vi "Forebrain.vi"() -> ()   [LabVIEW 2012]
doc: "This VI contrains the Forebrain within the Olin Robot Architecture. It must be run first to load the appropriate mission definition files. It contains a finite state machine built around a tabbed Operator interface that will guide an operator through the startup, run shutdown mission sequence. After running it, run the Midbrain and Hindbrain VIS."
panel:
  out "current MDF":T1(array[cluster])=[{"Status"=enum."Current", "x"=516.0, "y"=516.0, "z"=0.0, "Vel"=3.0, "Dwell Time"=0.0, "BehCom"=enum."Manual Mode", "X1"=0.0, "Y1"=0.0, "X2"=0.0, "Y2"=0.0}, {"Status"=enum."Future", "x"=0.0, "y"=0.0, "z"=0.0, "Vel"=0.0, "Dwell Time"=0.0, "BehCom"=enum."Tug Off", "X1"=0.0, "Y1"=0.0, "X2"=0.0, "Y2"=0.0}, {"Status"=enum."Future", "x"=0.0, "y"=0.0, "z"=0.0, "Vel"=0.0, "Dwell Time"=0.0, "BehCom"=enum."Tug Off", "X1"=0.0, "Y1"=0.0, "X2"=0.0, "Y2"=0.0}, {"Status"=enum."Future", "x"=0.0, "y"=0.0, "z"=0.0, "Vel"=0.0, "Dwell Time"=0.0, "BehCom"=enum."Tug Off", "X1"=0.0, "Y1"=0.0, "X2"=0.0, "Y2"=0.0}, {"Status"=enum."Future", "x"=0.0, "y"=0.0, "z"=0.0, "Vel"=0.0, "Dwell Time"=0.0, "BehCom"=enum."Tug Off", "X1"=0.0, "Y1"=0.0, "X2"=0.0, "Y2"=0.0}, {"Status"=enum."Future", "x"=0.0, "y"=0.0, "z"=0.0, "Vel"=0.0, "Dwell Time"=0.0, "BehCom"=enum."Tug Off", "X1"=0.0, "Y1"=0.0, "X2"=0.0, "Y2"=0.0}, {"Status"=enum."Future", "x"=0.0, "y"=0.0, "z"=0.0, "Vel"=0.0, "Dwell Time"=0.0, "BehCom"=enum."Tug Off", "X1"=0.0, "Y1"=0.0, "X2"=0.0, "Y2"=0.0}, {"Status"=enum."Future", "x"=0.0, "y"=0.0, "z"=0.0, "Vel"=0.0, "Dwell Time"=0.0, "BehCom"=enum."Tug Off", "X1"=0.0, "Y1"=0.0, "X2"=0.0, "Y2"=0.0}, {"Status"=enum."Future", "x"=0.0, "y"=0.0, "z"=0.0, "Vel"=0.0, "Dwell Time"=0.0, "BehCom"=enum."Tug Off", "X1"=0.0, "Y1"=0.0, "X2"=0.0, "Y2"=0.0}, {"Status"=enum."Future", "x"=0.0, "y"=0.0, "z"=0.0, "Vel"=0.0, "Dwell Time"=0.0, "BehCom"=enum."Tug Off", "X1"=0.0, "Y1"=0.0, "X2"=0.0, "Y2"=0.0}, {"Status"=enum."Future", "x"=0.0, "y"=0.0, "z"=0.0, "Vel"=0.0, "Dwell Time"=0.0, "BehCom"=enum."Tug Off", "X1"=0.0, "Y1"=0.0, "X2"=0.0, "Y2"=0.0}, {"Status"=enum."Future", "x"=0.0, "y"=0.0, "z"=0.0, "Vel"=0.0, "Dwell Time"=0.0, "BehCom"=enum."Tug Off", "X1"=0.0, "Y1"=0.0, "X2"=0.0, "Y2"=0.0}, {"Status"=enum."Future", "x"=0.0, "y"=0.0, "z"=0.0, "Vel"=0.0, "Dwell Time"=0.0, "BehCom"=enum."Tug Off", "X1"=0.0, "Y1"=0.0, "X2"=0.0, "Y2"=0.0}, {"Status"=enum."Future", "x"=0.0, "y"=0.0, "z"=0.0, "Vel"=0.0, "Dwell Time"=0.0, "BehCom"=enum."Tug Off", "X1"=0.0, "Y1"=0.0, "X2"=0.0, "Y2"=0.0}, {"Status"=enum."Future", "x"=0.0, "y"=0.0, "z"=0.0, "Vel"=0.0, "Dwell Time"=0.0, "BehCom"=enum."Tug Off", "X1"=0.0, "Y1"=0.0, "X2"=0.0, "Y2"=0.0}, {"Status"=enum."Future", "x"=0.0, "y"=0.0, "z"=0.0, "Vel"=0.0, "Dwell Time"=0.0, "BehCom"=enum."Tug Off", "X1"=0.0, "Y1"=0.0, "X2"=0.0, "Y2"=0.0}, {"Status"=enum."Future", "x"=0.0, "y"=0.0, "z"=0.0, "Vel"=0.0, "Dwell Time"=0.0, "BehCom"=enum."Tug Off", "X1"=0.0, "Y1"=0.0, "X2"=0.0, "Y2"=0.0}, {"Status"=enum."Future", "x"=0.0, "y"=0.0, "z"=0.0, "Vel"=0.0, "Dwell Time"=0.0, "BehCom"=enum."Tug Off", "X1"=0.0, "Y1"=0.0, "X2"=0.0, "Y2"=0.0}, {"Status"=enum."Future", "x"=0.0, "y"=0.0, "z"=0.0, "Vel"=0.0, "Dwell Time"=0.0, "BehCom"=enum."Tug Off", "X1"=0.0, "Y1"=0.0, "X2"=0.0, "Y2"=0.0}, {"Status"=enum."Future", "x"=0.0, "y"=0.0, "z"=0.0, "Vel"=0.0, "Dwell Time"=0.0, "BehCom"=enum."Tug Off", "X1"=0.0, "Y1"=0.0, "X2"=0.0, "Y2"=0.0}, {"Status"=enum."Future", "x"=0.0, "y"=0.0, "z"=0.0, "Vel"=0.0, "Dwell Time"=0.0, "BehCom"=enum."Tug Off", "X1"=0.0, "Y1"=0.0, "X2"=0.0, "Y2"=0.0}, {"Status"=enum."Future", "x"=0.0, "y"=0.0, "z"=0.0, "Vel"=0.0, "Dwell Time"=0.0, "BehCom"=enum."Tug Off", "X1"=0.0, "Y1"=0.0, "X2"=0.0, "Y2"=0.0}, {"Status"=enum."Future", "x"=0.0, "y"=0.0, "z"=0.0, "Vel"=0.0, "Dwell Time"=0.0, "BehCom"=enum."Tug Off", "X1"=0.0, "Y1"=0.0, "X2"=0.0, "Y2"=0.0}, {"Status"=enum."Future", "x"=0.0, "y"=0.0, "z"=0.0, "Vel"=0.0, "Dwell Time"=0.0, "BehCom"=enum."Tug Off", "X1"=0.0, "Y1"=0.0, "X2"=0.0, "Y2"=0.0}, {"Status"=enum."Future", "x"=0.0, "y"=0.0, "z"=0.0, "Vel"=0.0, "Dwell Time"=0.0, "BehCom"=enum."Tug Off", "X1"=0.0, "Y1"=0.0, "X2"=0.0, "Y2"=0.0}, {"Status"=enum."Future", "x"=0.0, "y"=0.0, "z"=0.0, "Vel"=0.0, "Dwell Time"=0.0, "BehCom"=enum."Tug Off", "X1"=0.0, "Y1"=0.0, "X2"=0.0, "Y2"=0.0}, {"Status"=enum."Future", "x"=0.0, "y"=0.0, "z"=0.0, "Vel"=0.0, "Dwell Time"=0.0, "BehCom"=enum."Tug Off", "X1"=0.0, "Y1"=0.0, "X2"=0.0, "Y2"=0.0}, {"Status"=enum."Future", "x"=0.0, "y"=0.0, "z"=0.0, "Vel"=0.0, "Dwell Time"=0.0, "BehCom"=enum."Tug Off", "X1"=0.0, "Y1"=0.0, "X2"=0.0, "Y2"=0.0}, {"Status"=enum."Future", "x"=0.0, "y"=0.0, "z"=0.0, "Vel"=0.0, "Dwell Time"=0.0, "BehCom"=enum."Tug Off", "X1"=0.0, "Y1"=0.0, "X2"=0.0, "Y2"=0.0}, {"Status"=enum."Future", "x"=0.0, "y"=0.0, "z"=0.0, "Vel"=0.0, "Dwell Time"=0.0, "BehCom"=enum."Tug Off", "X1"=0.0, "Y1"=0.0, "X2"=0.0, "Y2"=0.0}]
  out "Original MDF":T1(array[cluster])=[{"Status"=enum."Current", "x"=516.0, "y"=516.0, "z"=0.0, "Vel"=3.0, "Dwell Time"=0.0, "BehCom"=enum."Manual Mode", "X1"=0.0, "Y1"=0.0, "X2"=0.0, "Y2"=0.0}, {"Status"=enum."Future", "x"=0.0, "y"=0.0, "z"=0.0, "Vel"=0.0, "Dwell Time"=0.0, "BehCom"=enum."Tug Off", "X1"=0.0, "Y1"=0.0, "X2"=0.0, "Y2"=0.0}, {"Status"=enum."Future", "x"=0.0, "y"=0.0, "z"=0.0, "Vel"=0.0, "Dwell Time"=0.0, "BehCom"=enum."Tug Off", "X1"=0.0, "Y1"=0.0, "X2"=0.0, "Y2"=0.0}, {"Status"=enum."Future", "x"=0.0, "y"=0.0, "z"=0.0, "Vel"=0.0, "Dwell Time"=0.0, "BehCom"=enum."Tug Off", "X1"=0.0, "Y1"=0.0, "X2"=0.0, "Y2"=0.0}, {"Status"=enum."Future", "x"=0.0, "y"=0.0, "z"=0.0, "Vel"=0.0, "Dwell Time"=0.0, "BehCom"=enum."Tug Off", "X1"=0.0, "Y1"=0.0, "X2"=0.0, "Y2"=0.0}, {"Status"=enum."Future", "x"=0.0, "y"=0.0, "z"=0.0, "Vel"=0.0, "Dwell Time"=0.0, "BehCom"=enum."Tug Off", "X1"=0.0, "Y1"=0.0, "X2"=0.0, "Y2"=0.0}, {"Status"=enum."Future", "x"=0.0, "y"=0.0, "z"=0.0, "Vel"=0.0, "Dwell Time"=0.0, "BehCom"=enum."Tug Off", "X1"=0.0, "Y1"=0.0, "X2"=0.0, "Y2"=0.0}, {"Status"=enum."Future", "x"=0.0, "y"=0.0, "z"=0.0, "Vel"=0.0, "Dwell Time"=0.0, "BehCom"=enum."Tug Off", "X1"=0.0, "Y1"=0.0, "X2"=0.0, "Y2"=0.0}, {"Status"=enum."Future", "x"=0.0, "y"=0.0, "z"=0.0, "Vel"=0.0, "Dwell Time"=0.0, "BehCom"=enum."Tug Off", "X1"=0.0, "Y1"=0.0, "X2"=0.0, "Y2"=0.0}, {"Status"=enum."Future", "x"=0.0, "y"=0.0, "z"=0.0, "Vel"=0.0, "Dwell Time"=0.0, "BehCom"=enum."Tug Off", "X1"=0.0, "Y1"=0.0, "X2"=0.0, "Y2"=0.0}, {"Status"=enum."Future", "x"=0.0, "y"=0.0, "z"=0.0, "Vel"=0.0, "Dwell Time"=0.0, "BehCom"=enum."Tug Off", "X1"=0.0, "Y1"=0.0, "X2"=0.0, "Y2"=0.0}, {"Status"=enum."Future", "x"=0.0, "y"=0.0, "z"=0.0, "Vel"=0.0, "Dwell Time"=0.0, "BehCom"=enum."Tug Off", "X1"=0.0, "Y1"=0.0, "X2"=0.0, "Y2"=0.0}, {"Status"=enum."Future", "x"=0.0, "y"=0.0, "z"=0.0, "Vel"=0.0, "Dwell Time"=0.0, "BehCom"=enum."Tug Off", "X1"=0.0, "Y1"=0.0, "X2"=0.0, "Y2"=0.0}, {"Status"=enum."Future", "x"=0.0, "y"=0.0, "z"=0.0, "Vel"=0.0, "Dwell Time"=0.0, "BehCom"=enum."Tug Off", "X1"=0.0, "Y1"=0.0, "X2"=0.0, "Y2"=0.0}, {"Status"=enum."Future", "x"=0.0, "y"=0.0, "z"=0.0, "Vel"=0.0, "Dwell Time"=0.0, "BehCom"=enum."Tug Off", "X1"=0.0, "Y1"=0.0, "X2"=0.0, "Y2"=0.0}, {"Status"=enum."Future", "x"=0.0, "y"=0.0, "z"=0.0, "Vel"=0.0, "Dwell Time"=0.0, "BehCom"=enum."Tug Off", "X1"=0.0, "Y1"=0.0, "X2"=0.0, "Y2"=0.0}, {"Status"=enum."Future", "x"=0.0, "y"=0.0, "z"=0.0, "Vel"=0.0, "Dwell Time"=0.0, "BehCom"=enum."Tug Off", "X1"=0.0, "Y1"=0.0, "X2"=0.0, "Y2"=0.0}, {"Status"=enum."Future", "x"=0.0, "y"=0.0, "z"=0.0, "Vel"=0.0, "Dwell Time"=0.0, "BehCom"=enum."Tug Off", "X1"=0.0, "Y1"=0.0, "X2"=0.0, "Y2"=0.0}, {"Status"=enum."Future", "x"=0.0, "y"=0.0, "z"=0.0, "Vel"=0.0, "Dwell Time"=0.0, "BehCom"=enum."Tug Off", "X1"=0.0, "Y1"=0.0, "X2"=0.0, "Y2"=0.0}, {"Status"=enum."Future", "x"=0.0, "y"=0.0, "z"=0.0, "Vel"=0.0, "Dwell Time"=0.0, "BehCom"=enum."Tug Off", "X1"=0.0, "Y1"=0.0, "X2"=0.0, "Y2"=0.0}, {"Status"=enum."Future", "x"=0.0, "y"=0.0, "z"=0.0, "Vel"=0.0, "Dwell Time"=0.0, "BehCom"=enum."Tug Off", "X1"=0.0, "Y1"=0.0, "X2"=0.0, "Y2"=0.0}, {"Status"=enum."Future", "x"=0.0, "y"=0.0, "z"=0.0, "Vel"=0.0, "Dwell Time"=0.0, "BehCom"=enum."Tug Off", "X1"=0.0, "Y1"=0.0, "X2"=0.0, "Y2"=0.0}, {"Status"=enum."Future", "x"=0.0, "y"=0.0, "z"=0.0, "Vel"=0.0, "Dwell Time"=0.0, "BehCom"=enum."Tug Off", "X1"=0.0, "Y1"=0.0, "X2"=0.0, "Y2"=0.0}, {"Status"=enum."Future", "x"=0.0, "y"=0.0, "z"=0.0, "Vel"=0.0, "Dwell Time"=0.0, "BehCom"=enum."Tug Off", "X1"=0.0, "Y1"=0.0, "X2"=0.0, "Y2"=0.0}, {"Status"=enum."Future", "x"=0.0, "y"=0.0, "z"=0.0, "Vel"=0.0, "Dwell Time"=0.0, "BehCom"=enum."Tug Off", "X1"=0.0, "Y1"=0.0, "X2"=0.0, "Y2"=0.0}, {"Status"=enum."Future", "x"=0.0, "y"=0.0, "z"=0.0, "Vel"=0.0, "Dwell Time"=0.0, "BehCom"=enum."Tug Off", "X1"=0.0, "Y1"=0.0, "X2"=0.0, "Y2"=0.0}, {"Status"=enum."Future", "x"=0.0, "y"=0.0, "z"=0.0, "Vel"=0.0, "Dwell Time"=0.0, "BehCom"=enum."Tug Off", "X1"=0.0, "Y1"=0.0, "X2"=0.0, "Y2"=0.0}, {"Status"=enum."Future", "x"=0.0, "y"=0.0, "z"=0.0, "Vel"=0.0, "Dwell Time"=0.0, "BehCom"=enum."Tug Off", "X1"=0.0, "Y1"=0.0, "X2"=0.0, "Y2"=0.0}, {"Status"=enum."Future", "x"=0.0, "y"=0.0, "z"=0.0, "Vel"=0.0, "Dwell Time"=0.0, "BehCom"=enum."Tug Off", "X1"=0.0, "Y1"=0.0, "X2"=0.0, "Y2"=0.0}, {"Status"=enum."Future", "x"=0.0, "y"=0.0, "z"=0.0, "Vel"=0.0, "Dwell Time"=0.0, "BehCom"=enum."Tug Off", "X1"=0.0, "Y1"=0.0, "X2"=0.0, "Y2"=0.0}]
  out "No. of Waypoints":i32=30
  in  "A Midbrain?":bool
  in  "Manuel\nLocation":bool
  in  "Fake Heading":i32
  in  "Fake X":i32
  in  "Fake Y":i32
  out "return count":u32=11
  out "error out":errorcluster
  in  "error in 2":errorcluster
  out "Desired \nVelocity":i16
  out "Local\nHeading":i16
  out "Ycurrent":dbl=744.0 format="%#_3g"
  out "Xcurrent":dbl=683.0 format="%#_3g"
  out "Ystart":dbl=400.0
  out "Xstart":dbl=500.0
  in  "error in":errorcluster
  out "Robot Live":bool=TRUE
  in  "E-Stop":bool
  in  "Tab":T2(tab)=enum."PlanMission"
  out "MissionTime (Min)":dbl(knob)=1.6143843173980712 scale=0.0..10.0
  out "LidarDist":i16=800
  out "IR Index":i32
  out "BatteryLevel":dbl(slide)=7.0 scale=6.0..9.0
  out "String Received":string="{800,13,48520}<13,10,13>"
  out "Send String":string="[AGHBAAAAA]"
  in  "VISA resource name":refnum<visa-resource-name>="COM7"
  in  "Mode":i16=1 min=0 max=99 step=1
  in  "Desired Vel":i16(slide) scale=-9.0..9.0
  in  "Local Head":i16(slide) scale=-180.0..180.0
  out "StartMissionMap":picture
  out "MapDARCheck":picture
  in  "RunRobot":bool=TRUE
  in  "Tug letter":string="T"
  out "Tug X":i32=683
  out "Tug Y":i32=744
  out "Tug H":i32=220
  out "BS Time Out?":bool
  out "Buoy locations":cluster{"regular expression":string, i32, i32}[](array[cluster])=[{"regular expression"="A", 229, 772}, {"regular expression"="B", 828, 412}, {"regular expression"="C", 634, 873}, {"regular expression"="D", 229, 278}]
  out "Valid ?":bool
  out "Battery\nVolts":i16=7000
  out "Base Station data rec'd":string="$,G,-1,-1,-1,T,-1,-1,-1,P,-1,-1,-1,L,-1,-1,-1,A,229,772,B,828,412,C,634,873,D,229,278,S,23,43,27\r"
  out "udp rate":bool=TRUE
  out "CollisionWarning":bool
  out "DebugMapDAR":picture
  in  "MapDAR Control":T3={"NumberOfBeams"=180, "SensorRange"=500.0, "Noise (0.1 to 1)"=0.0} {"Noise (0.1 to 1)" min=0.0 max=1.0 step=0.1; "SensorRange" min=500.0 max=1500.0 step=100.0; "NumberOfBeams" min=36 max=360 step=2}
  out "MapDAR Data (r:pixel b:degrees)":cluster{"Range":dbl, "Bearing":dbl}[](array[cluster])
  in  "Stop DebugSENSE":bool
  out "MissionMap":picture
  out "Tug position":T4
  out "initialized MDF":T1(array[cluster])=[{"Status"=enum."Current", "x"=516.0, "y"=516.0, "z"=0.0, "Vel"=3.0, "Dwell Time"=0.0, "BehCom"=enum."Manual Mode", "X1"=0.0, "Y1"=0.0, "X2"=0.0, "Y2"=0.0}, {"Status"=enum."Future", "x"=0.0, "y"=0.0, "z"=0.0, "Vel"=0.0, "Dwell Time"=0.0, "BehCom"=enum."Tug Off", "X1"=0.0, "Y1"=0.0, "X2"=0.0, "Y2"=0.0}, {"Status"=enum."Future", "x"=0.0, "y"=0.0, "z"=0.0, "Vel"=0.0, "Dwell Time"=0.0, "BehCom"=enum."Tug Off", "X1"=0.0, "Y1"=0.0, "X2"=0.0, "Y2"=0.0}, {"Status"=enum."Future", "x"=0.0, "y"=0.0, "z"=0.0, "Vel"=0.0, "Dwell Time"=0.0, "BehCom"=enum."Tug Off", "X1"=0.0, "Y1"=0.0, "X2"=0.0, "Y2"=0.0}, {"Status"=enum."Future", "x"=0.0, "y"=0.0, "z"=0.0, "Vel"=0.0, "Dwell Time"=0.0, "BehCom"=enum."Tug Off", "X1"=0.0, "Y1"=0.0, "X2"=0.0, "Y2"=0.0}, {"Status"=enum."Future", "x"=0.0, "y"=0.0, "z"=0.0, "Vel"=0.0, "Dwell Time"=0.0, "BehCom"=enum."Tug Off", "X1"=0.0, "Y1"=0.0, "X2"=0.0, "Y2"=0.0}, {"Status"=enum."Future", "x"=0.0, "y"=0.0, "z"=0.0, "Vel"=0.0, "Dwell Time"=0.0, "BehCom"=enum."Tug Off", "X1"=0.0, "Y1"=0.0, "X2"=0.0, "Y2"=0.0}, {"Status"=enum."Future", "x"=0.0, "y"=0.0, "z"=0.0, "Vel"=0.0, "Dwell Time"=0.0, "BehCom"=enum."Tug Off", "X1"=0.0, "Y1"=0.0, "X2"=0.0, "Y2"=0.0}, {"Status"=enum."Future", "x"=0.0, "y"=0.0, "z"=0.0, "Vel"=0.0, "Dwell Time"=0.0, "BehCom"=enum."Tug Off", "X1"=0.0, "Y1"=0.0, "X2"=0.0, "Y2"=0.0}, {"Status"=enum."Future", "x"=0.0, "y"=0.0, "z"=0.0, "Vel"=0.0, "Dwell Time"=0.0, "BehCom"=enum."Tug Off", "X1"=0.0, "Y1"=0.0, "X2"=0.0, "Y2"=0.0}, {"Status"=enum."Future", "x"=0.0, "y"=0.0, "z"=0.0, "Vel"=0.0, "Dwell Time"=0.0, "BehCom"=enum."Tug Off", "X1"=0.0, "Y1"=0.0, "X2"=0.0, "Y2"=0.0}, {"Status"=enum."Future", "x"=0.0, "y"=0.0, "z"=0.0, "Vel"=0.0, "Dwell Time"=0.0, "BehCom"=enum."Tug Off", "X1"=0.0, "Y1"=0.0, "X2"=0.0, "Y2"=0.0}, {"Status"=enum."Future", "x"=0.0, "y"=0.0, "z"=0.0, "Vel"=0.0, "Dwell Time"=0.0, "BehCom"=enum."Tug Off", "X1"=0.0, "Y1"=0.0, "X2"=0.0, "Y2"=0.0}, {"Status"=enum."Future", "x"=0.0, "y"=0.0, "z"=0.0, "Vel"=0.0, "Dwell Time"=0.0, "BehCom"=enum."Tug Off", "X1"=0.0, "Y1"=0.0, "X2"=0.0, "Y2"=0.0}, {"Status"=enum."Future", "x"=0.0, "y"=0.0, "z"=0.0, "Vel"=0.0, "Dwell Time"=0.0, "BehCom"=enum."Tug Off", "X1"=0.0, "Y1"=0.0, "X2"=0.0, "Y2"=0.0}, {"Status"=enum."Future", "x"=0.0, "y"=0.0, "z"=0.0, "Vel"=0.0, "Dwell Time"=0.0, "BehCom"=enum."Tug Off", "X1"=0.0, "Y1"=0.0, "X2"=0.0, "Y2"=0.0}, {"Status"=enum."Future", "x"=0.0, "y"=0.0, "z"=0.0, "Vel"=0.0, "Dwell Time"=0.0, "BehCom"=enum."Tug Off", "X1"=0.0, "Y1"=0.0, "X2"=0.0, "Y2"=0.0}, {"Status"=enum."Future", "x"=0.0, "y"=0.0, "z"=0.0, "Vel"=0.0, "Dwell Time"=0.0, "BehCom"=enum."Tug Off", "X1"=0.0, "Y1"=0.0, "X2"=0.0, "Y2"=0.0}, {"Status"=enum."Future", "x"=0.0, "y"=0.0, "z"=0.0, "Vel"=0.0, "Dwell Time"=0.0, "BehCom"=enum."Tug Off", "X1"=0.0, "Y1"=0.0, "X2"=0.0, "Y2"=0.0}, {"Status"=enum."Future", "x"=0.0, "y"=0.0, "z"=0.0, "Vel"=0.0, "Dwell Time"=0.0, "BehCom"=enum."Tug Off", "X1"=0.0, "Y1"=0.0, "X2"=0.0, "Y2"=0.0}, {"Status"=enum."Future", "x"=0.0, "y"=0.0, "z"=0.0, "Vel"=0.0, "Dwell Time"=0.0, "BehCom"=enum."Tug Off", "X1"=0.0, "Y1"=0.0, "X2"=0.0, "Y2"=0.0}, {"Status"=enum."Future", "x"=0.0, "y"=0.0, "z"=0.0, "Vel"=0.0, "Dwell Time"=0.0, "BehCom"=enum."Tug Off", "X1"=0.0, "Y1"=0.0, "X2"=0.0, "Y2"=0.0}, {"Status"=enum."Future", "x"=0.0, "y"=0.0, "z"=0.0, "Vel"=0.0, "Dwell Time"=0.0, "BehCom"=enum."Tug Off", "X1"=0.0, "Y1"=0.0, "X2"=0.0, "Y2"=0.0}, {"Status"=enum."Future", "x"=0.0, "y"=0.0, "z"=0.0, "Vel"=0.0, "Dwell Time"=0.0, "BehCom"=enum."Tug Off", "X1"=0.0, "Y1"=0.0, "X2"=0.0, "Y2"=0.0}, {"Status"=enum."Future", "x"=0.0, "y"=0.0, "z"=0.0, "Vel"=0.0, "Dwell Time"=0.0, "BehCom"=enum."Tug Off", "X1"=0.0, "Y1"=0.0, "X2"=0.0, "Y2"=0.0}, {"Status"=enum."Future", "x"=0.0, "y"=0.0, "z"=0.0, "Vel"=0.0, "Dwell Time"=0.0, "BehCom"=enum."Tug Off", "X1"=0.0, "Y1"=0.0, "X2"=0.0, "Y2"=0.0}, {"Status"=enum."Future", "x"=0.0, "y"=0.0, "z"=0.0, "Vel"=0.0, "Dwell Time"=0.0, "BehCom"=enum."Tug Off", "X1"=0.0, "Y1"=0.0, "X2"=0.0, "Y2"=0.0}, {"Status"=enum."Future", "x"=0.0, "y"=0.0, "z"=0.0, "Vel"=0.0, "Dwell Time"=0.0, "BehCom"=enum."Tug Off", "X1"=0.0, "Y1"=0.0, "X2"=0.0, "Y2"=0.0}, {"Status"=enum."Future", "x"=0.0, "y"=0.0, "z"=0.0, "Vel"=0.0, "Dwell Time"=0.0, "BehCom"=enum."Tug Off", "X1"=0.0, "Y1"=0.0, "X2"=0.0, "Y2"=0.0}, {"Status"=enum."Future", "x"=0.0, "y"=0.0, "z"=0.0, "Vel"=0.0, "Dwell Time"=0.0, "BehCom"=enum."Tug Off", "X1"=0.0, "Y1"=0.0, "X2"=0.0, "Y2"=0.0}]
  out "Way Point Index":i32
  in  "WhereAmI?FromBase":T5={"T"=1.5970837354660035, "X"=683.0, "Y"=744.0, "Direction"=220.0}
  out "(xr,yr)":cluster{"X":dbl, "Y":dbl}={"X"=197.0, "Y"=316.0}
  in  "RobotPosition":T4 {"xrobot" min=0.0 max=1177.0 step=10.0; "yrobot" min=0.0 max=850.0 step=10.0; "heading" min=0.0 max=7.0 step=0.1}
  out "WhatAroundMeMap?":cluster{"T":dbl, "Range":dbl, "Bearing":dbl}[](array[cluster])=[{"T"=1.613952883084615, "Range"=500.7064053008593, "Bearing"=89.99998125548201}, {"T"=1.613952883084615, "Range"=500.5978288083754, "Bearing"=87.99998125593866}, {"T"=1.613952883084615, "Range"=500.21663447161455, "Bearing"=85.99998125639532}, {"T"=1.613952883084615, "Range"=500.95231100174755, "Bearing"=83.999981256852}, {"T"=1.613952883084615, "Range"=501.00810550574045, "Bearing"=81.99998125730865}, {"T"=1.613952883084615, "Range"=500.443083561566, "Bearing"=79.9999812577653}, {"T"=1.613952883084615, "Range"=500.32154501238114, "Bearing"=77.99998125822196}, {"T"=1.613952883084615, "Range"=499.6891722644295, "Bearing"=75.99998125867863}, {"T"=1.613952883084615, "Range"=499.6096835149916, "Bearing"=73.99998125913528}, {"T"=1.613952883084615, "Range"=499.1091515696598, "Bearing"=71.99998125959193}, {"T"=1.613952883084615, "Range"=498.21454583521466, "Bearing"=69.9999812600486}, {"T"=1.613952883084615, "Range"=497.9900262589242, "Bearing"=67.99998126050525}, {"T"=1.613952883084615, "Range"=497.4147592132127, "Bearing"=65.9999812609619}, {"T"=1.613952883084615, "Range"=497.5582636361386, "Bearing"=63.999981261418576}, {"T"=1.613952883084615, "Range"=497.3581605268189, "Bearing"=61.999981261875234}, {"T"=1.613952883084615, "Range"=497.89381867996866, "Bearing"=59.9999812623319}, {"T"=1.613952883084615, "Range"=498.05085856753595, "Bearing"=57.99998126278856}, {"T"=1.613952883084615, "Range"=497.77182452894067, "Bearing"=55.99998126324521}, {"T"=1.613952883084615, "Range"=498.15786754668255, "Bearing"=53.99998126370187}, {"T"=1.613952883084615, "Range"=499.19636381215463, "Bearing"=51.99998126415853}, {"T"=1.613952883084615, "Range"=499.6330940653848, "Bearing"=49.999981264615194}, {"T"=1.613952883084615, "Range"=499.3440349654286, "Bearing"=47.999981265071845}, {"T"=1.613952883084615, "Range"=499.4893176352856, "Bearing"=45.99998126552851}, {"T"=1.613952883084615, "Range"=500.0173205915729, "Bearing"=43.99998126598517}, {"T"=1.613952883084615, "Range"=499.4791512349587, "Bearing"=41.99998126644182}, {"T"=1.613952883084615, "Range"=482.93682012184183, "Bearing"=39.99998126689849}, {"T"=1.613952883084615, "Range"=468.09918320629475, "Bearing"=37.99998126735514}, {"T"=1.613952883084615, "Range"=454.3790677497674, "Bearing"=35.999981267811805}, {"T"=1.613952883084615, "Range"=441.73316028028927, "Bearing"=33.99998126826846}, {"T"=1.613952883084615, "Range"=430.1181473258901, "Bearing"=31.99998126872512}, {"T"=1.613952883084615, "Range"=419.49071541459995, "Bearing"=29.999981269181788}, {"T"=1.613952883084615, "Range"=409.80755107444776, "Bearing"=27.999981269638443}, {"T"=1.613952883084615, "Range"=401.0253408334638, "Bearing"=25.9999812700951}, {"T"=1.613952883084615, "Range"=393.1007712196775, "Bearing"=23.999981270551757}, {"T"=1.613952883084615, "Range"=385.99052876111864, "Bearing"=21.999981271008412}, {"T"=1.613952883084615, "Range"=379.65129998581676, "Bearing"=19.99998127146508}, {"T"=1.613952883084615, "Range"=374.03977142180156, "Bearing"=17.999981271921737}, {"T"=1.613952883084615, "Range"=369.1126295971028, "Bearing"=15.999981272378394}, {"T"=1.613952883084615, "Range"=364.8265610397501, "Bearing"=13.99998127283505}, {"T"=1.613952883084615, "Range"=361.1382522777731, "Bearing"=11.999981273291718}, {"T"=1.613952883084615, "Range"=358.00438983920145, "Bearing"=9.999981273748375}, {"T"=1.613952883084615, "Range"=355.3816602520649, "Bearing"=7.999981274205032}, {"T"=1.613952883084615, "Range"=353.22675004439304, "Bearing"=5.999981274661688}, {"T"=1.613952883084615, "Range"=351.49634574421566, "Bearing"=3.9999812751183446}, {"T"=1.613952883084615, "Range"=350.1471338795622, "Bearing"=1.9999812755750135}, {"T"=1.613952883084615, "Range"=349.13580097846256, "Bearing"=-1.872396833026647e-05}, {"T"=1.613952883084615, "Range"=348.4190335689462, "Bearing"=-2.000018723511674}, {"T"=1.613952883084615, "Range"=348.0130409259428, "Bearing"=-4.0000187230550175}, {"T"=1.613952883084615, "Range"=348.5159307988174, "Bearing"=-6.000018722598361}, {"T"=1.613952883084615, "Range"=345.2719100021574, "Bearing"=-8.000018722141693}, {"T"=1.613952883084615, "Range"=339.2763368608847, "Bearing"=-10.000018721685036}, {"T"=1.613952883084615, "Range"=333.5659980898058, "Bearing"=-12.000018721228379}, {"T"=1.613952883084615, "Range"=328.91456786552607, "Bearing"=-14.000018720771724}, {"T"=1.613952883084615, "Range"=328.1797162019266, "Bearing"=-16.000018720315055}, {"T"=1.613952883084615, "Range"=326.5495177558285, "Bearing"=-18.0000187198584}, {"T"=1.613952883084615, "Range"=323.2450066703523, "Bearing"=-20.00001871940174}, {"T"=1.613952883084615, "Range"=321.3770172581106, "Bearing"=-22.000018718945086}, {"T"=1.613952883084615, "Range"=321.1705289415094, "Bearing"=-24.00001871848843}, {"T"=1.613952883084615, "Range"=317.808161867162, "Bearing"=-26.00001871803177}, {"T"=1.613952883084615, "Range"=316.10046941909906, "Bearing"=-28.000018717575117}, {"T"=1.613952883084615, "Range"=314.80727311533974, "Bearing"=-30.000018717118433}, {"T"=1.613952883084615, "Range"=316.1498591489302, "Bearing"=-32.00001871666178}, {"T"=1.613952883084615, "Range"=316.82540716219296, "Bearing"=-34.00001871620512}, {"T"=1.613952883084615, "Range"=316.4612195595032, "Bearing"=-36.00001871574847}, {"T"=1.613952883084615, "Range"=315.88754898053077, "Bearing"=-38.00001871529181}, {"T"=1.613952883084615, "Range"=306.65805152928766, "Bearing"=-40.00001871483515}, {"T"=1.613952883084615, "Range"=313.69553669692516, "Bearing"=-42.0000187143785}, {"T"=1.613952883084615, "Range"=312.25531682956637, "Bearing"=-44.00001871392184}, {"T"=1.613952883084615, "Range"=311.92268520354264, "Bearing"=-46.00001871346518}, {"T"=1.613952883084615, "Range"=298.5464332493932, "Bearing"=-48.0000187130085}, {"T"=1.613952883084615, "Range"=304.1652200959302, "Bearing"=-50.00001871255184}, {"T"=1.613952883084615, "Range"=302.7613976136267, "Bearing"=-52.00001871209519}, {"T"=1.613952883084615, "Range"=301.9420825510875, "Bearing"=-54.00001871163853}, {"T"=1.613952883084615, "Range"=301.07174408003493, "Bearing"=-56.00001871118187}, {"T"=1.613952883084615, "Range"=300.51223892347906, "Bearing"=-58.00001871072522}, {"T"=1.613952883084615, "Range"=300.2863564776341, "Bearing"=-60.00001871026856}, {"T"=1.613952883084615, "Range"=296.90119773931013, "Bearing"=-62.000018709811904}, {"T"=1.613952883084615, "Range"=295.1877811420984, "Bearing"=-64.00001870935525}, {"T"=1.613952883084615, "Range"=293.919874937399, "Bearing"=-66.00001870889857}, {"T"=1.613952883084615, "Range"=294.2548309699896, "Bearing"=-68.00001870844191}, {"T"=1.613952883084615, "Range"=297.0274025795303, "Bearing"=-70.00001870798526}, {"T"=1.613952883084615, "Range"=298.8996820027432, "Bearing"=-72.0000187075286}, {"T"=1.613952883084615, "Range"=301.69020555606016, "Bearing"=-74.00001870707194}, {"T"=1.613952883084615, "Range"=300.3772692009894, "Bearing"=-76.0000187066153}, {"T"=1.613952883084615, "Range"=297.453358358428, "Bearing"=-78.00001870615863}, {"T"=1.613952883084615, "Range"=294.9815906263283, "Bearing"=-80.00001870570198}, {"T"=1.613952883084615, "Range"=292.9230625807171, "Bearing"=-82.00001870524532}, {"T"=1.613952883084615, "Range"=291.2388707976212, "Bearing"=-84.00001870478864}, {"T"=1.613952883084615, "Range"=289.8901118530667, "Bearing"=-86.00001870433198}, {"T"=1.613952883084615, "Range"=288.837882323081, "Bearing"=-88.00001870387533}, {"T"=1.613952883084615, "Range"=288.0432787836905, "Bearing"=-90.00001870341868}, {"T"=1.613952883084615, "Range"=287.4673978109218, "Bearing"=-92.00001870296201}, {"T"=1.613952883084615, "Range"=286.9528050111057, "Bearing"=-94.00001870250536}, {"T"=1.613952883084615, "Range"=287.43197266969776, "Bearing"=-96.0000187020487}, {"T"=1.613952883084615, "Range"=288.10366852050265, "Bearing"=-98.00001870159204}, {"T"=1.613952883084615, "Range"=289.00556992349334, "Bearing"=-100.00001870113539}, {"T"=1.613952883084615, "Range"=290.175354238645, "Bearing"=-102.00001870067874}, {"T"=1.613952883084615, "Range"=291.65069882593093, "Bearing"=-104.00001870022204}, {"T"=1.613952883084615, "Range"=293.4692810453258, "Bearing"=-106.00001869976539}, {"T"=1.613952883084615, "Range"=295.6687782568041, "Bearing"=-108.00001869930874}, {"T"=1.613952883084615, "Range"=298.28686782033975, "Bearing"=-110.00001869885207}, {"T"=1.613952883084615, "Range"=301.36122709590654, "Bearing"=-112.00001869839542}, {"T"=1.613952883084615, "Range"=304.9295334434793, "Bearing"=-114.00001869793877}, {"T"=1.613952883084615, "Range"=309.0294642230314, "Bearing"=-116.0000186974821}, {"T"=1.613952883084615, "Range"=313.69869679453797, "Bearing"=-118.00001869702545}, {"T"=1.613952883084615, "Range"=318.9749085179729, "Bearing"=-120.0000186965688}, {"T"=1.613952883084615, "Range"=324.89577675331026, "Bearing"=-122.00001869611212}, {"T"=1.613952883084615, "Range"=331.49897886052395, "Bearing"=-124.00001869565546}, {"T"=1.613952883084615, "Range"=338.8221921995884, "Bearing"=-126.0000186951988}, {"T"=1.613952883084615, "Range"=346.9030941304783, "Bearing"=-128.00001869474215}, {"T"=1.613952883084615, "Range"=355.77936201316726, "Bearing"=-130.0000186942855}, {"T"=1.613952883084615, "Range"=365.488673207629, "Bearing"=-132.00001869382882}, {"T"=1.613952883084615, "Range"=376.068705073839, "Bearing"=-134.00001869337217}, {"T"=1.613952883084615, "Range"=387.5571349717704, "Bearing"=-136.00001869291552}, {"T"=1.613952883084615, "Range"=399.99164026139835, "Bearing"=-138.00001869245887}, {"T"=1.613952883084615, "Range"=415.2488179443076, "Bearing"=-140.0000186920022}, {"T"=1.613952883084615, "Range"=432.0480630156488, "Bearing"=-142.00001869154556}, {"T"=1.613952883084615, "Range"=449.4140711573864, "Bearing"=-144.00001869108888}, {"T"=1.613952883084615, "Range"=468.67903150964327, "Bearing"=-146.00001869063223}, {"T"=1.613952883084615, "Range"=491.04868052532584, "Bearing"=-148.00001869017555}, {"T"=1.613952883084615, "Range"=500.7379168649637, "Bearing"=-150.00001868971887}, {"T"=1.613952883084615, "Range"=501.1150247987179, "Bearing"=-152.00001868926225}, {"T"=1.613952883084615, "Range"=500.9459085440803, "Bearing"=-154.00001868880557}, {"T"=1.613952883084615, "Range"=500.31705856405466, "Bearing"=-156.00001868834894}, {"T"=1.613952883084615, "Range"=500.40721219153363, "Bearing"=-158.00001868789226}, {"T"=1.613952883084615, "Range"=500.11732628421515, "Bearing"=-160.0000186874356}, {"T"=1.613952883084615, "Range"=500.56381193891644, "Bearing"=-162.00001868697893}, {"T"=1.613952883084615, "Range"=500.6621072239231, "Bearing"=-164.0000186865223}, {"T"=1.613952883084615, "Range"=501.4777594461184, "Bearing"=-166.00001868606563}, {"T"=1.613952883084615, "Range"=501.93518972623264, "Bearing"=-168.00001868560895}, {"T"=1.613952883084615, "Range"=502.02435784260916, "Bearing"=-170.00001868515233}, {"T"=1.613952883084615, "Range"=502.7514379824436, "Bearing"=-172.00001868469562}, {"T"=1.613952883084615, "Range"=504.0669107962158, "Bearing"=-174.000018684239}, {"T"=1.613952883084615, "Range"=503.8831963997854, "Bearing"=-176.00001868378232}, {"T"=1.613952883084615, "Range"=504.19619581855125, "Bearing"=-178.0000186833257}, {"T"=1.613952883084615, "Range"=504.94448256176963, "Bearing"=-180.000018682869}, {"T"=1.613952883084615, "Range"=505.0554348530047, "Bearing"=-182.0000186824124}, {"T"=1.613952883084615, "Range"=496.41823890366686, "Bearing"=-184.00001868195568}, {"T"=1.613952883084615, "Range"=497.17595663872595, "Bearing"=-186.000018681499}, {"T"=1.613952883084615, "Range"=497.2716409874367, "Bearing"=-188.00001868104238}, {"T"=1.613952883084615, "Range"=496.7619777677218, "Bearing"=-190.0000186805857}, {"T"=1.613952883084615, "Range"=496.70150077719956, "Bearing"=-192.00001868012907}, {"T"=1.613952883084615, "Range"=496.1409251456773, "Bearing"=-194.0000186796724}, {"T"=1.613952883084615, "Range"=496.1344022617209, "Bearing"=-196.00001867921574}, {"T"=1.613952883084615, "Range"=495.7128986210873, "Bearing"=-198.00001867875906}, {"T"=1.613952883084615, "Range"=494.90102773923013, "Bearing"=-200.00001867830244}, {"T"=1.613952883084615, "Range"=494.7538871067457, "Bearing"=-202.00001867784576}, {"T"=1.613952883084615, "Range"=494.2555091349043, "Bearing"=-204.00001867738908}, {"T"=1.613952883084615, "Range"=494.4667738446001, "Bearing"=-206.00001867693246}, {"T"=1.613952883084615, "Range"=494.3303090337049, "Bearing"=-208.00001867647578}, {"T"=1.613952883084615, "Range"=494.9172911971745, "Bearing"=-210.00001867601912}, {"T"=1.613952883084615, "Range"=495.11865325571955, "Bearing"=-212.00001867556244}, {"T"=1.613952883084615, "Range"=494.8758863289303, "Bearing"=-214.00001867510582}, {"T"=1.613952883084615, "Range"=495.2826450984663, "Bearing"=-216.00001867464914}, {"T"=1.613952883084615, "Range"=496.32559248403226, "Bearing"=-218.00001867419252}, {"T"=1.613952883084615, "Range"=496.7570686208392, "Bearing"=-220.00001867373584}, {"T"=1.613952883084615, "Range"=496.4533541216331, "Bearing"=-222.00001867327916}, {"T"=1.613952883084615, "Range"=496.5677267586635, "Bearing"=-224.0000186728225}, {"T"=1.613952883084615, "Range"=497.04883389602224, "Bearing"=-226.00001867236583}, {"T"=1.613952883084615, "Range"=496.4566589484559, "Bearing"=-228.0000186719092}, {"T"=1.613952883084615, "Range"=495.0738096506831, "Bearing"=-230.0000186714525}, {"T"=1.613952883084615, "Range"=495.41186174096254, "Bearing"=-232.00001867099593}, {"T"=1.613952883084615, "Range"=494.70891988254516, "Bearing"=-234.00001867053925}, {"T"=1.613952883084615, "Range"=494.39293134677246, "Bearing"=-236.00001867008254}, {"T"=1.613952883084615, "Range"=493.2964675530977, "Bearing"=-238.00001866962586}, {"T"=1.613952883084615, "Range"=492.743531886521, "Bearing"=-240.00001866916918}, {"T"=1.613952883084615, "Range"=492.76440117319817, "Bearing"=-242.0000186687126}, {"T"=1.613952883084615, "Range"=492.2497142278405, "Bearing"=-244.00001866825593}, {"T"=1.613952883084615, "Range"=491.2870241972635, "Bearing"=-246.00001866779925}, {"T"=1.613952883084615, "Range"=491.03532772819244, "Bearing"=-248.00001866734257}, {"T"=1.613952883084615, "Range"=490.41671623618834, "Bearing"=-250.00001866688598}, {"T"=1.613952883084615, "Range"=490.5270902361183, "Bearing"=-252.0000186664293}, {"T"=1.613952883084615, "Range"=490.3038460099097, "Bearing"=-254.00001866597262}, {"T"=1.613952883084615, "Range"=490.7912350266706, "Bearing"=-256.00001866551594}, {"T"=1.613952883084615, "Range"=490.9364756365754, "Bearing"=-258.00001866505926}, {"T"=1.613952883084615, "Range"=490.73071702175594, "Bearing"=-260.0000186646027}, {"T"=1.613952883084615, "Range"=491.15763660782994, "Bearing"=-262.000018664146}, {"T"=1.613952883084615, "Range"=492.16766896531664, "Bearing"=-264.00001866368933}, {"T"=1.613952883084615, "Range"=491.72232297221865, "Bearing"=-266.00001866323265}, {"T"=1.613952883084615, "Range"=491.7700582034097, "Bearing"=-268.00001866277603}]
  out "WayPointAct":dbl[](array[numeric])=[3.0, 2.9961677067438224, 2.984700174911875, 2.9656850740521508, 2.9392672792150147, 2.9056470328726154, 2.86507741748726, 2.81786118335041, 2.764346987303046, 2.7049251076850824, 2.6400227091403, 2.5700987375578945, 2.4956385303397677, 2.417148230268107, 2.335149092482053, 2.2501717734741127, 2.162750688650594, 2.073418520972506, 1.9827009576490586, 1.8911117249731209, 1.799147983371763, 1.7072861358207037, 1.6159780931776804, 1.5256480299715354, 1.4366896539851954, 1.3494640028286715, 1.2642977708359453, 1.1814821602417387, 1.101272241881713, 1.0238868027667969, 0.949508650933647, 0.8782853420621721, 0.8103302875394018, 0.7457241999674091, 0.6845168295621473, 0.6267289434429443, 0.5723544994169317, 0.5213629664451154, 0.4737017454453488, 0.4292986463362949, 0.3880643801395689, 0.34989502841258924, 0.31467445615781287, 0.2822766385217612, 0.25256787594081404, 0.22540887679839858, 0.20065669102771216, 0.17816648233440954, 0.15779313074612872, 0.1393926609550322, 0.12282349535390816, 0.10794753373756093, 0.09463106432393806, 0.08274551303060372, 0.07216803981984514, 0.06278199240781046, 0.05447722873604609, 0.04715032035107638, 0.04070464925821259, 0.03505041094265283, 0.030104536119876957, 0.025790543425487283, 0.02203833471939763, 0.018783943997251317, 0.01596925010817775, 0.013541662605209824, 0.011453789132785996, 0.009663091811480107, 0.008131539136753404, 0.006825258985905336, 0.00571419744183336, 0.004771787306625294, 0.003974629402151323, 0.0033021890455026998, 0.002736509448503557, 0.0022619432244394303, 0.0018649026914454804, 0.001533629238867161, 0.0012579816671993017, 0.0010292431197532965, 0.0008399459900791054, 0.0006837140079736222, 0.0005551205729677751, 0.0004495623117568568, 0.0003631467794615238, 0.0002925931984343286, 0.00023514512742274233, 0.00018849397351299943, 0.00015071229508849994, 0.0001201958921788532]
  out "SteerAngle":dbl=45.0
  in  "Tab Control":enum32{"Mission 1", "Mission 2", "Mission 3"}(tab)
  in  "Mission 1":T6(array[cluster])=[{"X"=516.0, "Y"=516.0, "Vel"=3.0, "Select Your Behavior"=enum."Manual Mode", "X1"=0.0, "X2"=0.0, "Y2"=0.0, "Y1"=0.0}, {"X"=0.0, "Y"=0.0, "Vel"=0.0, "Select Your Behavior"=enum."Tug Off", "X1"=0.0, "X2"=0.0, "Y2"=0.0, "Y1"=0.0}, {"X"=0.0, "Y"=0.0, "Vel"=0.0, "Select Your Behavior"=enum."Tug Off", "X1"=0.0, "X2"=0.0, "Y2"=0.0, "Y1"=0.0}, {"X"=0.0, "Y"=0.0, "Vel"=0.0, "Select Your Behavior"=enum."Tug Off", "X1"=0.0, "X2"=0.0, "Y2"=0.0, "Y1"=0.0}, {"X"=0.0, "Y"=0.0, "Vel"=0.0, "Select Your Behavior"=enum."Tug Off", "X1"=0.0, "X2"=0.0, "Y2"=0.0, "Y1"=0.0}, {"X"=0.0, "Y"=0.0, "Vel"=0.0, "Select Your Behavior"=enum."Tug Off", "X1"=0.0, "X2"=0.0, "Y2"=0.0, "Y1"=0.0}, {"X"=0.0, "Y"=0.0, "Vel"=0.0, "Select Your Behavior"=enum."Tug Off", "X1"=0.0, "X2"=0.0, "Y2"=0.0, "Y1"=0.0}, {"X"=0.0, "Y"=0.0, "Vel"=0.0, "Select Your Behavior"=enum."Tug Off", "X1"=0.0, "X2"=0.0, "Y2"=0.0, "Y1"=0.0}, {"X"=0.0, "Y"=0.0, "Vel"=0.0, "Select Your Behavior"=enum."Tug Off", "X1"=0.0, "X2"=0.0, "Y2"=0.0, "Y1"=0.0}, {"X"=0.0, "Y"=0.0, "Vel"=0.0, "Select Your Behavior"=enum."Tug Off", "X1"=0.0, "X2"=0.0, "Y2"=0.0, "Y1"=0.0}, {"X"=0.0, "Y"=0.0, "Vel"=0.0, "Select Your Behavior"=enum."Tug Off", "X1"=0.0, "X2"=0.0, "Y2"=0.0, "Y1"=0.0}, {"X"=0.0, "Y"=0.0, "Vel"=0.0, "Select Your Behavior"=enum."Tug Off", "X1"=0.0, "X2"=0.0, "Y2"=0.0, "Y1"=0.0}, {"X"=0.0, "Y"=0.0, "Vel"=0.0, "Select Your Behavior"=enum."Tug Off", "X1"=0.0, "X2"=0.0, "Y2"=0.0, "Y1"=0.0}, {"X"=0.0, "Y"=0.0, "Vel"=0.0, "Select Your Behavior"=enum."Tug Off", "X1"=0.0, "X2"=0.0, "Y2"=0.0, "Y1"=0.0}, {"X"=0.0, "Y"=0.0, "Vel"=0.0, "Select Your Behavior"=enum."Tug Off", "X1"=0.0, "X2"=0.0, "Y2"=0.0, "Y1"=0.0}, {"X"=0.0, "Y"=0.0, "Vel"=0.0, "Select Your Behavior"=enum."Tug Off", "X1"=0.0, "X2"=0.0, "Y2"=0.0, "Y1"=0.0}, {"X"=0.0, "Y"=0.0, "Vel"=0.0, "Select Your Behavior"=enum."Tug Off", "X1"=0.0, "X2"=0.0, "Y2"=0.0, "Y1"=0.0}, {"X"=0.0, "Y"=0.0, "Vel"=0.0, "Select Your Behavior"=enum."Tug Off", "X1"=0.0, "X2"=0.0, "Y2"=0.0, "Y1"=0.0}, {"X"=0.0, "Y"=0.0, "Vel"=0.0, "Select Your Behavior"=enum."Tug Off", "X1"=0.0, "X2"=0.0, "Y2"=0.0, "Y1"=0.0}, {"X"=0.0, "Y"=0.0, "Vel"=0.0, "Select Your Behavior"=enum."Tug Off", "X1"=0.0, "X2"=0.0, "Y2"=0.0, "Y1"=0.0}, {"X"=0.0, "Y"=0.0, "Vel"=0.0, "Select Your Behavior"=enum."Tug Off", "X1"=0.0, "X2"=0.0, "Y2"=0.0, "Y1"=0.0}, {"X"=0.0, "Y"=0.0, "Vel"=0.0, "Select Your Behavior"=enum."Tug Off", "X1"=0.0, "X2"=0.0, "Y2"=0.0, "Y1"=0.0}, {"X"=0.0, "Y"=0.0, "Vel"=0.0, "Select Your Behavior"=enum."Tug Off", "X1"=0.0, "X2"=0.0, "Y2"=0.0, "Y1"=0.0}, {"X"=0.0, "Y"=0.0, "Vel"=0.0, "Select Your Behavior"=enum."Tug Off", "X1"=0.0, "X2"=0.0, "Y2"=0.0, "Y1"=0.0}, {"X"=0.0, "Y"=0.0, "Vel"=0.0, "Select Your Behavior"=enum."Tug Off", "X1"=0.0, "X2"=0.0, "Y2"=0.0, "Y1"=0.0}, {"X"=0.0, "Y"=0.0, "Vel"=0.0, "Select Your Behavior"=enum."Tug Off", "X1"=0.0, "X2"=0.0, "Y2"=0.0, "Y1"=0.0}, {"X"=0.0, "Y"=0.0, "Vel"=0.0, "Select Your Behavior"=enum."Tug Off", "X1"=0.0, "X2"=0.0, "Y2"=0.0, "Y1"=0.0}, {"X"=0.0, "Y"=0.0, "Vel"=0.0, "Select Your Behavior"=enum."Tug Off", "X1"=0.0, "X2"=0.0, "Y2"=0.0, "Y1"=0.0}, {"X"=0.0, "Y"=0.0, "Vel"=0.0, "Select Your Behavior"=enum."Tug Off", "X1"=0.0, "X2"=0.0, "Y2"=0.0, "Y1"=0.0}, {"X"=0.0, "Y"=0.0, "Vel"=0.0, "Select Your Behavior"=enum."Tug Off", "X1"=0.0, "X2"=0.0, "Y2"=0.0, "Y1"=0.0}, {"X"=0.0, "Y"=0.0, "Vel"=0.0, "Select Your Behavior"=enum."Tug Off", "X1"=0.0, "X2"=0.0, "Y2"=0.0, "Y1"=0.0}]
  in  "Mission 2":T6(array[cluster])=[{"X"=0.0, "Y"=0.0, "Vel"=0.0, "Select Your Behavior"=enum."Tug Off", "X1"=0.0, "X2"=0.0, "Y2"=0.0, "Y1"=0.0}, {"X"=0.0, "Y"=0.0, "Vel"=0.0, "Select Your Behavior"=enum."Tug Off", "X1"=0.0, "X2"=0.0, "Y2"=0.0, "Y1"=0.0}, {"X"=0.0, "Y"=0.0, "Vel"=0.0, "Select Your Behavior"=enum."Tug Off", "X1"=0.0, "X2"=0.0, "Y2"=0.0, "Y1"=0.0}, {"X"=0.0, "Y"=0.0, "Vel"=0.0, "Select Your Behavior"=enum."Tug Off", "X1"=0.0, "X2"=0.0, "Y2"=0.0, "Y1"=0.0}, {"X"=0.0, "Y"=0.0, "Vel"=0.0, "Select Your Behavior"=enum."Tug Off", "X1"=0.0, "X2"=0.0, "Y2"=0.0, "Y1"=0.0}, {"X"=0.0, "Y"=0.0, "Vel"=0.0, "Select Your Behavior"=enum."Tug Off", "X1"=0.0, "X2"=0.0, "Y2"=0.0, "Y1"=0.0}, {"X"=0.0, "Y"=0.0, "Vel"=0.0, "Select Your Behavior"=enum."Tug Off", "X1"=0.0, "X2"=0.0, "Y2"=0.0, "Y1"=0.0}, {"X"=0.0, "Y"=0.0, "Vel"=0.0, "Select Your Behavior"=enum."Tug Off", "X1"=0.0, "X2"=0.0, "Y2"=0.0, "Y1"=0.0}, {"X"=0.0, "Y"=0.0, "Vel"=0.0, "Select Your Behavior"=enum."Tug Off", "X1"=0.0, "X2"=0.0, "Y2"=0.0, "Y1"=0.0}, {"X"=0.0, "Y"=0.0, "Vel"=0.0, "Select Your Behavior"=enum."Tug Off", "X1"=0.0, "X2"=0.0, "Y2"=0.0, "Y1"=0.0}, {"X"=0.0, "Y"=0.0, "Vel"=0.0, "Select Your Behavior"=enum."Tug Off", "X1"=0.0, "X2"=0.0, "Y2"=0.0, "Y1"=0.0}, {"X"=0.0, "Y"=0.0, "Vel"=0.0, "Select Your Behavior"=enum."Tug Off", "X1"=0.0, "X2"=0.0, "Y2"=0.0, "Y1"=0.0}, {"X"=0.0, "Y"=0.0, "Vel"=0.0, "Select Your Behavior"=enum."Tug Off", "X1"=0.0, "X2"=0.0, "Y2"=0.0, "Y1"=0.0}, {"X"=0.0, "Y"=0.0, "Vel"=0.0, "Select Your Behavior"=enum."Tug Off", "X1"=0.0, "X2"=0.0, "Y2"=0.0, "Y1"=0.0}, {"X"=0.0, "Y"=0.0, "Vel"=0.0, "Select Your Behavior"=enum."Tug Off", "X1"=0.0, "X2"=0.0, "Y2"=0.0, "Y1"=0.0}, {"X"=0.0, "Y"=0.0, "Vel"=0.0, "Select Your Behavior"=enum."Tug Off", "X1"=0.0, "X2"=0.0, "Y2"=0.0, "Y1"=0.0}, {"X"=0.0, "Y"=0.0, "Vel"=0.0, "Select Your Behavior"=enum."Tug Off", "X1"=0.0, "X2"=0.0, "Y2"=0.0, "Y1"=0.0}, {"X"=0.0, "Y"=0.0, "Vel"=0.0, "Select Your Behavior"=enum."Tug Off", "X1"=0.0, "X2"=0.0, "Y2"=0.0, "Y1"=0.0}, {"X"=0.0, "Y"=0.0, "Vel"=0.0, "Select Your Behavior"=enum."Tug Off", "X1"=0.0, "X2"=0.0, "Y2"=0.0, "Y1"=0.0}, {"X"=0.0, "Y"=0.0, "Vel"=0.0, "Select Your Behavior"=enum."Tug Off", "X1"=0.0, "X2"=0.0, "Y2"=0.0, "Y1"=0.0}, {"X"=0.0, "Y"=0.0, "Vel"=0.0, "Select Your Behavior"=enum."Tug Off", "X1"=0.0, "X2"=0.0, "Y2"=0.0, "Y1"=0.0}, {"X"=0.0, "Y"=0.0, "Vel"=0.0, "Select Your Behavior"=enum."Tug Off", "X1"=0.0, "X2"=0.0, "Y2"=0.0, "Y1"=0.0}, {"X"=0.0, "Y"=0.0, "Vel"=0.0, "Select Your Behavior"=enum."Tug Off", "X1"=0.0, "X2"=0.0, "Y2"=0.0, "Y1"=0.0}, {"X"=0.0, "Y"=0.0, "Vel"=0.0, "Select Your Behavior"=enum."Tug Off", "X1"=0.0, "X2"=0.0, "Y2"=0.0, "Y1"=0.0}, {"X"=0.0, "Y"=0.0, "Vel"=0.0, "Select Your Behavior"=enum."Tug Off", "X1"=0.0, "X2"=0.0, "Y2"=0.0, "Y1"=0.0}, {"X"=0.0, "Y"=0.0, "Vel"=0.0, "Select Your Behavior"=enum."Tug Off", "X1"=0.0, "X2"=0.0, "Y2"=0.0, "Y1"=0.0}, {"X"=0.0, "Y"=0.0, "Vel"=0.0, "Select Your Behavior"=enum."Tug Off", "X1"=0.0, "X2"=0.0, "Y2"=0.0, "Y1"=0.0}, {"X"=0.0, "Y"=0.0, "Vel"=0.0, "Select Your Behavior"=enum."Tug Off", "X1"=0.0, "X2"=0.0, "Y2"=0.0, "Y1"=0.0}, {"X"=0.0, "Y"=0.0, "Vel"=0.0, "Select Your Behavior"=enum."Tug Off", "X1"=0.0, "X2"=0.0, "Y2"=0.0, "Y1"=0.0}, {"X"=0.0, "Y"=0.0, "Vel"=0.0, "Select Your Behavior"=enum."Tug Off", "X1"=0.0, "X2"=0.0, "Y2"=0.0, "Y1"=0.0}, {"X"=0.0, "Y"=0.0, "Vel"=0.0, "Select Your Behavior"=enum."Tug Off", "X1"=0.0, "X2"=0.0, "Y2"=0.0, "Y1"=0.0}]
  in  "Mission 3":T6(array[cluster])=[{"X"=0.0, "Y"=0.0, "Vel"=0.0, "Select Your Behavior"=enum."Tug Off", "X1"=0.0, "X2"=0.0, "Y2"=0.0, "Y1"=0.0}, {"X"=0.0, "Y"=0.0, "Vel"=0.0, "Select Your Behavior"=enum."Tug Off", "X1"=0.0, "X2"=0.0, "Y2"=0.0, "Y1"=0.0}, {"X"=0.0, "Y"=0.0, "Vel"=0.0, "Select Your Behavior"=enum."Tug Off", "X1"=0.0, "X2"=0.0, "Y2"=0.0, "Y1"=0.0}, {"X"=0.0, "Y"=0.0, "Vel"=0.0, "Select Your Behavior"=enum."Tug Off", "X1"=0.0, "X2"=0.0, "Y2"=0.0, "Y1"=0.0}, {"X"=0.0, "Y"=0.0, "Vel"=0.0, "Select Your Behavior"=enum."Tug Off", "X1"=0.0, "X2"=0.0, "Y2"=0.0, "Y1"=0.0}, {"X"=0.0, "Y"=0.0, "Vel"=0.0, "Select Your Behavior"=enum."Tug Off", "X1"=0.0, "X2"=0.0, "Y2"=0.0, "Y1"=0.0}, {"X"=0.0, "Y"=0.0, "Vel"=0.0, "Select Your Behavior"=enum."Tug Off", "X1"=0.0, "X2"=0.0, "Y2"=0.0, "Y1"=0.0}, {"X"=0.0, "Y"=0.0, "Vel"=0.0, "Select Your Behavior"=enum."Tug Off", "X1"=0.0, "X2"=0.0, "Y2"=0.0, "Y1"=0.0}, {"X"=0.0, "Y"=0.0, "Vel"=0.0, "Select Your Behavior"=enum."Tug Off", "X1"=0.0, "X2"=0.0, "Y2"=0.0, "Y1"=0.0}, {"X"=0.0, "Y"=0.0, "Vel"=0.0, "Select Your Behavior"=enum."Tug Off", "X1"=0.0, "X2"=0.0, "Y2"=0.0, "Y1"=0.0}, {"X"=0.0, "Y"=0.0, "Vel"=0.0, "Select Your Behavior"=enum."Tug Off", "X1"=0.0, "X2"=0.0, "Y2"=0.0, "Y1"=0.0}, {"X"=0.0, "Y"=0.0, "Vel"=0.0, "Select Your Behavior"=enum."Tug Off", "X1"=0.0, "X2"=0.0, "Y2"=0.0, "Y1"=0.0}, {"X"=0.0, "Y"=0.0, "Vel"=0.0, "Select Your Behavior"=enum."Tug Off", "X1"=0.0, "X2"=0.0, "Y2"=0.0, "Y1"=0.0}, {"X"=0.0, "Y"=0.0, "Vel"=0.0, "Select Your Behavior"=enum."Tug Off", "X1"=0.0, "X2"=0.0, "Y2"=0.0, "Y1"=0.0}, {"X"=0.0, "Y"=0.0, "Vel"=0.0, "Select Your Behavior"=enum."Tug Off", "X1"=0.0, "X2"=0.0, "Y2"=0.0, "Y1"=0.0}, {"X"=0.0, "Y"=0.0, "Vel"=0.0, "Select Your Behavior"=enum."Tug Off", "X1"=0.0, "X2"=0.0, "Y2"=0.0, "Y1"=0.0}, {"X"=0.0, "Y"=0.0, "Vel"=0.0, "Select Your Behavior"=enum."Tug Off", "X1"=0.0, "X2"=0.0, "Y2"=0.0, "Y1"=0.0}, {"X"=0.0, "Y"=0.0, "Vel"=0.0, "Select Your Behavior"=enum."Tug Off", "X1"=0.0, "X2"=0.0, "Y2"=0.0, "Y1"=0.0}, {"X"=0.0, "Y"=0.0, "Vel"=0.0, "Select Your Behavior"=enum."Tug Off", "X1"=0.0, "X2"=0.0, "Y2"=0.0, "Y1"=0.0}, {"X"=0.0, "Y"=0.0, "Vel"=0.0, "Select Your Behavior"=enum."Tug Off", "X1"=0.0, "X2"=0.0, "Y2"=0.0, "Y1"=0.0}, {"X"=0.0, "Y"=0.0, "Vel"=0.0, "Select Your Behavior"=enum."Tug Off", "X1"=0.0, "X2"=0.0, "Y2"=0.0, "Y1"=0.0}, {"X"=0.0, "Y"=0.0, "Vel"=0.0, "Select Your Behavior"=enum."Tug Off", "X1"=0.0, "X2"=0.0, "Y2"=0.0, "Y1"=0.0}, {"X"=0.0, "Y"=0.0, "Vel"=0.0, "Select Your Behavior"=enum."Tug Off", "X1"=0.0, "X2"=0.0, "Y2"=0.0, "Y1"=0.0}, {"X"=0.0, "Y"=0.0, "Vel"=0.0, "Select Your Behavior"=enum."Tug Off", "X1"=0.0, "X2"=0.0, "Y2"=0.0, "Y1"=0.0}, {"X"=0.0, "Y"=0.0, "Vel"=0.0, "Select Your Behavior"=enum."Tug Off", "X1"=0.0, "X2"=0.0, "Y2"=0.0, "Y1"=0.0}, {"X"=0.0, "Y"=0.0, "Vel"=0.0, "Select Your Behavior"=enum."Tug Off", "X1"=0.0, "X2"=0.0, "Y2"=0.0, "Y1"=0.0}, {"X"=0.0, "Y"=0.0, "Vel"=0.0, "Select Your Behavior"=enum."Tug Off", "X1"=0.0, "X2"=0.0, "Y2"=0.0, "Y1"=0.0}, {"X"=0.0, "Y"=0.0, "Vel"=0.0, "Select Your Behavior"=enum."Tug Off", "X1"=0.0, "X2"=0.0, "Y2"=0.0, "Y1"=0.0}, {"X"=0.0, "Y"=0.0, "Vel"=0.0, "Select Your Behavior"=enum."Tug Off", "X1"=0.0, "X2"=0.0, "Y2"=0.0, "Y1"=0.0}, {"X"=0.0, "Y"=0.0, "Vel"=0.0, "Select Your Behavior"=enum."Tug Off", "X1"=0.0, "X2"=0.0, "Y2"=0.0, "Y1"=0.0}, {"X"=0.0, "Y"=0.0, "Vel"=0.0, "Select Your Behavior"=enum."Tug Off", "X1"=0.0, "X2"=0.0, "Y2"=0.0, "Y1"=0.0}]
  out "MissionDefFile":picture
  in  "Exit Planning":bool
  out "BuildMDF":bool
  out "Send String to NXT":string="[AGHBAAAAA]"
  in  "Behavior Command":T7(ring)=enum."Manual Mode"
  out "CollisionLight":bool
  out "Where? Manual":T5={"T"=2.448372713724772, "X"=197.0, "Y"=316.0, "Direction"=25.0}
  out "ActManual":bool
  in  "Manual Heading":i16(knob)=1 min=-179 max=180 step=5 scale=180.0..-180.0
  out "MWhat?":bool=TRUE
  out "Where? 2":bool
  out "How? 2":bool
  in  "ManualModeStop":bool
  out "ManualModeMapDAR":picture
  out "ManualMissionMap":picture
  out "Battery":dbl(slide)=7.0 scale=0.0..8.0
  in  "Manual Vel":dbl(slide) min=-6.0 max=6.0 step=1.0 scale=-6.0..6.0
  out "MissionTime":dbl(knob)=3.2816865841547647 scale=0.0..10.0
  out "Heading":cluster{dbl, dbl}(knob)={25.0, 1.0} scale=180.0..-179.0 scale format="%#_3g"
  out "Speed":i16(knob) scale=-6.0..6.0
  out "Current Behavior":T7(ring)=enum."Manual Mode"
  out "Robot Position":cluster{"X":dbl, "Y":dbl}={"X"=666.0, "Y"=560.0} {"X" format="%#_3g"; "Y" format="%#_3g"}
  out "Ready":bool=TRUE
  in  "Pause":bool
  in  "Rerun MDF":bool
  out "CollisionLight 2":bool
  out "Act":bool=TRUE
  out "Neo-C":bool=TRUE
  out "How?":bool=TRUE
  out "What?":bool
  out "A Heading":cluster{dbl, dbl}(knob)={-88.0, 45.0} scale=180.0..-180.0
  out "A Speed":dbl(knob)=3.0 scale=-9.0..9.0
  out "AutoBattery":dbl(slide)=7.0 scale=0.0..8.0
  out "AutoModeLIDAR":picture
  out "AutoMissionMap":picture
  in  "RunAutoMode":bool=TRUE
  out "MissionTimeAuto":dbl(knob)=1.5813821315765382 scale=0.0..60.0
  out "Where?":bool=TRUE
  # "To run\nrobot,\nclick\narrow\nabove\n\nRun Robot button must be on"
  # "Operation Directions\n\n1)Click on Startup&\nShutdown tab.\n2) Click on Run \nArrow on menubar.\nRun Forebrain,\nvis from the project\nexplorer.\n3) Select a mssion \nmap file when asked.\n4) Check robot is \nfully operational on\nStartup tab.\n5) Debug with debug\ntabs as required.\n6) Select ManualMode\ntab and test drive \nrobot.\n7) Select PlanMission\ntab and set up \nmission.\n8) Go to AutoMode\ntab and run mission."
  # "Turns off drive\nmotors"
  # "Enter Olin Test  Pool"
  # "Xbee Com Port"
  # "xBee\"Send String\" (mode, desired velocity, local heading)"
  # "(Type in Tug Letter  L T G P  (look at boat cradle)"
  # "Should be on to\nrun"
  # "BoatG,X,Y,H,BoatT,X,Y,H,BoatP,X,Y.H,BoatL,X,Y,H,BuoyA,X,Y,BuoyB,X,Y,BuoyC,X,Y,BuoyD,X,Y,Time(hours,Min,Sec)"
  # "To stop  program \nturn off here"
  # "Use this tab\nto explore\nLIDAR\ndata and \noperation"
  # "Set\nNumberOfBeams\nSensorRange\nNoise\nto\nview\nsimulated\nsensor\ndata"
  # "Turn Debug Sim \nto leave this\ntab--->"
  # "This tab will auto\nreturn to Startup \nin 2 seconds"
  # "Clean up interface and make more useful for debugging behaviors"
  # "Build out interface and make more useful for debugging act"
  # "This tab will auto\nreturn to Startup \nin 2 seconds"
  # "Directions:\n1) Select Robot Behavior for each mission leg.\n2) Select Robot Speed for leg.\n3) Click on robots current location for first waypoint.\n4) Hold down button and drag to next\nwaypoint. Click on next leg waypoint.\n5) Hold mouse button down and drag to \nnext waypoint. \n6) Click on next waypoint. Repeat for full mission.\n7) MDF will store up to 20 waypoints."
  # "Please Adjust Scroll Barrs in Tug Off Mode to Prevent  Extra Lines Being Drawn"
  # "If Go TO Waypoint:"
  # "If Gate"
  # "If Go TO Waypoint:"
  # "If Gate"
  # "If Go TO Waypoint:"
  # "If Gate"
  # "\"Send String\" (mode, desired velocity, local heading)"
  # "Press to stop and return to StartUp"
  # "Open MidBrain\nArbiter to see\nBrain Waves"
  # "AutoMode\nAutomatically \nReturns to \nStartUp Mode"
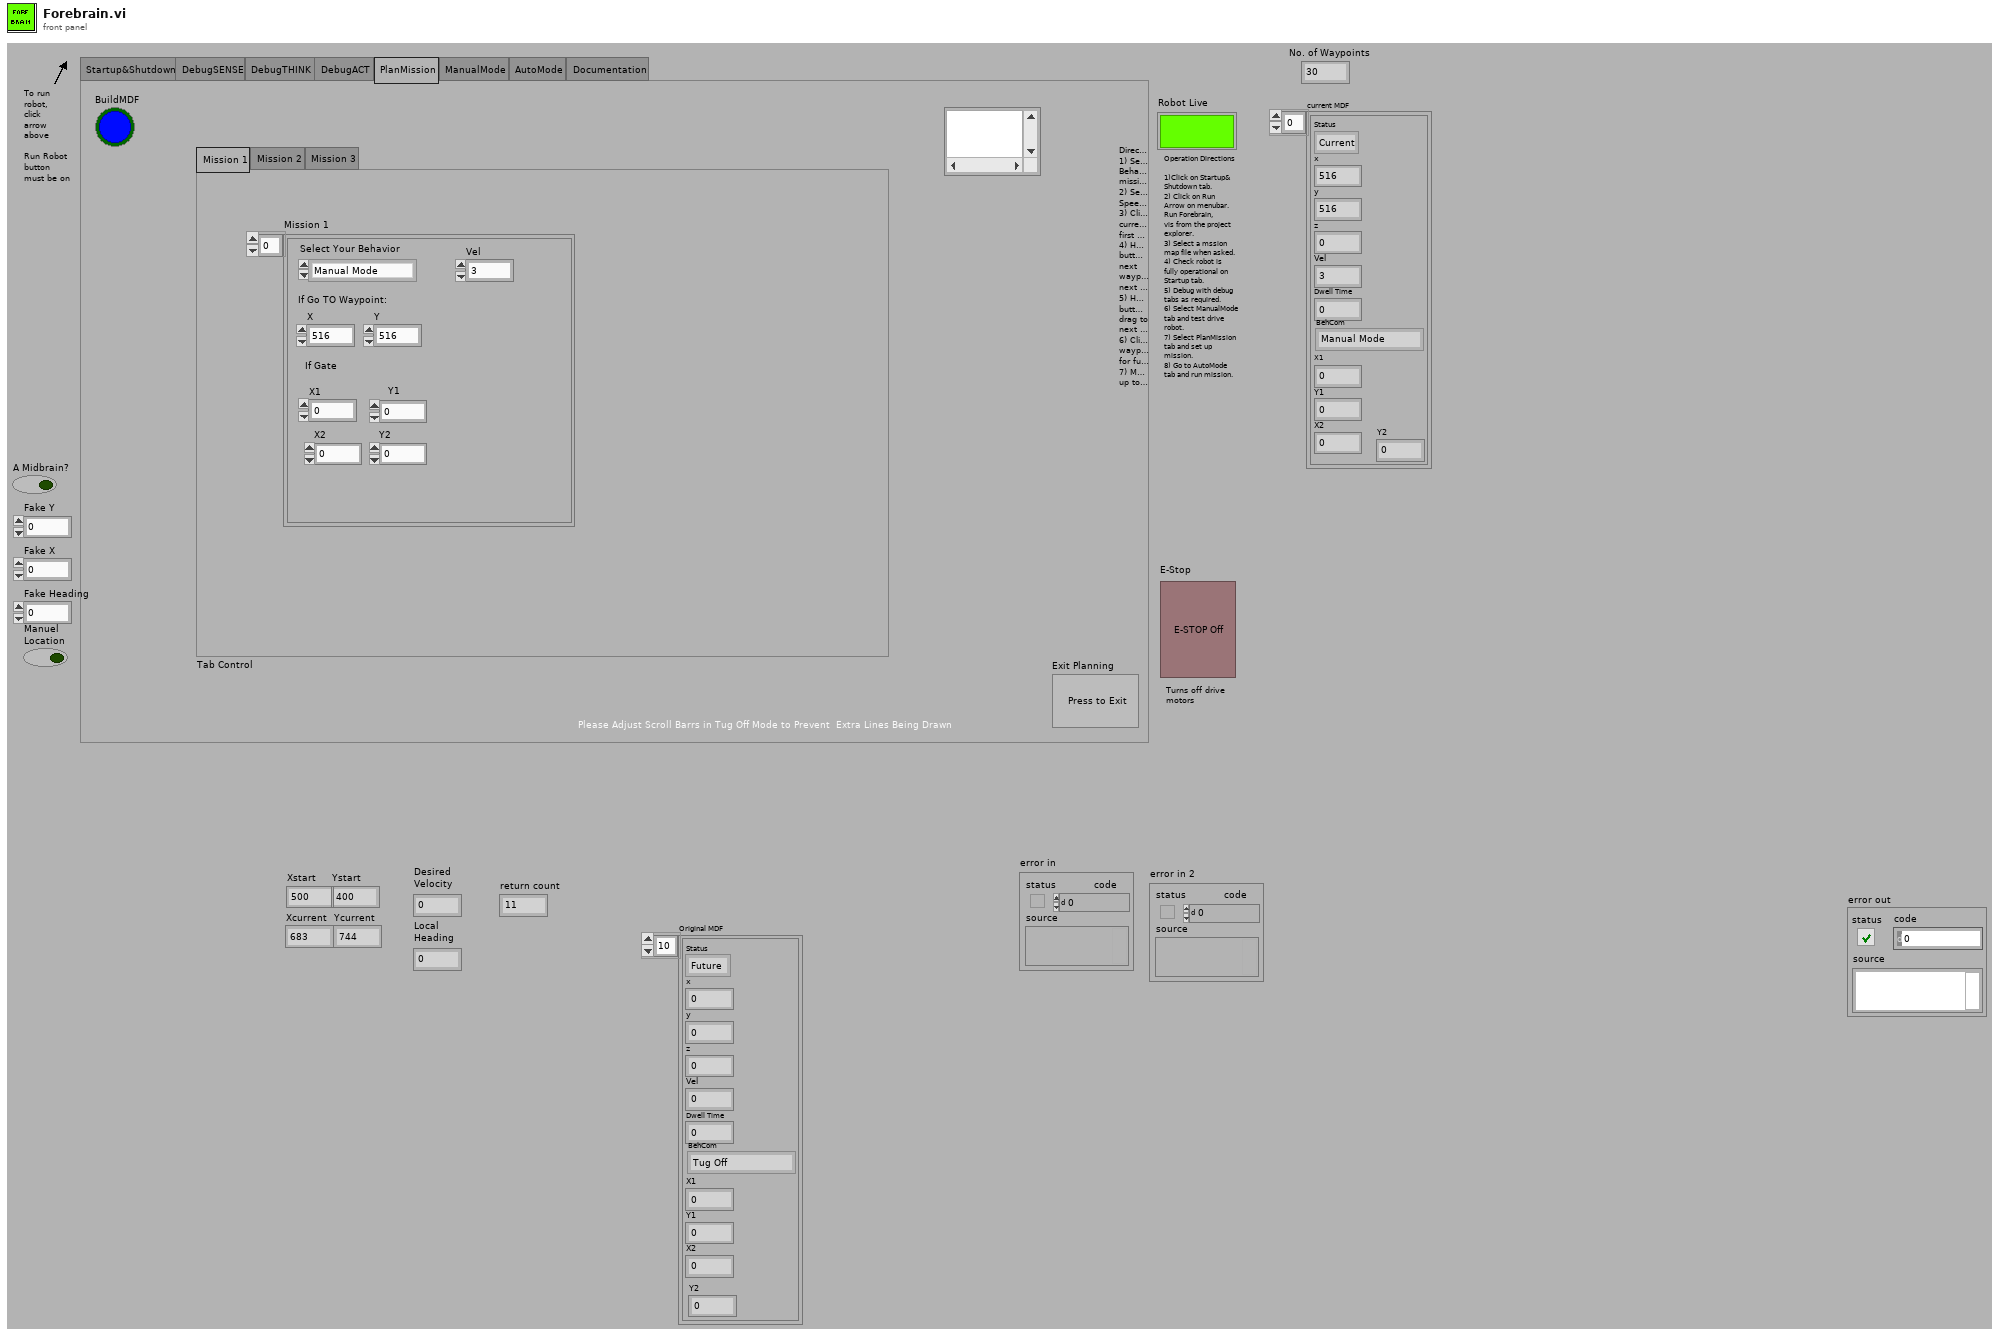
[diagram p1: front panel]
types:
  T1 = cluster{"Status":enum16{"Past", "Current", "Future"}, "x":dbl, "y":dbl, "z":dbl, "Vel":dbl, "Dwell Time":dbl, "BehCom":enum16{"Tug Off", "Manual Mode", "Goto WayPoint", "Back Up", "Gate", "Left Wall Follow", "Right Wall Follow", "Hunt"}, "X1":dbl, "Y1":dbl, "X2":dbl, "Y2":dbl}[]
  T2 = enum32{"Startup&Shutdown", "DebugSENSE", "DebugTHINK", "DebugACT", "PlanMission", "ManualMode", "AutoMode", "Documentation"}
  T3 = cluster{"NumberOfBeams":i32, "SensorRange":dbl, "Noise (0.1 to 1)":dbl}
  T4 = cluster{"xrobot":dbl, "yrobot":dbl, "heading":dbl}
  T5 = cluster{"T":dbl, "X":dbl, "Y":dbl, "Direction":dbl}
  T6 = cluster{"X":dbl, "Y":dbl, "Vel":dbl, "Select Your Behavior":enum16{"Tug Off", "Manual Mode", "Goto WayPoint", "Back Up", "Gate", "Left Wall Follow", "Right Wall Follow", "Hunt"}, "X1":dbl, "X2":dbl, "Y2":dbl, "Y1":dbl}[]
  T7 = enum16{"Tug Off", "Manual Mode", "Goto WayPoint", "Back Up", "Circle", "Left Wall Follow", "Right Wall Follow", "Hunt"}
  T8 = enum16{"Tug Off", "Manual Mode", "Goto WayPoint", "Back Up", "Gate", "Left Wall Follow", "Right Wall Follow", "Hunt"}
  T9 = cluster{"VelCom":dbl, "BehCom":enum16{"OpenFieldTransit", "P-WallFollow", "S-WallFollow", "LaneFollow", "ManualMode"}}
  T10 = typedef "IMAQ Image.ctl" = refnum<image>
  T11 = typedef "imagedata.ctl" = cluster{"image type":i32, "image depth":i32, "image":u8[], "mask":u8[], "colors":u32[], "Rectangle":cluster{"left":i16, "top":i16, "right":i16, "bottom":i16}}
  T12 = cluster{"regular expression":string, i32, i32, i32}
  T13 = cluster{dbl, "Fake X":i32, "Fake Y":i32, "Fake Heading":i32}
  T14 = cluster{"Status":enum16{"Past", "Current", "Future"}, "x":dbl, "y":dbl, "z":dbl, "Vel":dbl, "Dwell Time":dbl, "BehCom":enum16{"Tug Off", "Manual Mode", "Goto WayPoint", "Back Up", "Gate", "Left Wall Follow", "Right Wall Follow", "Hunt"}, "Expand1":dbl, "Expand2":dbl, "Expand3":dbl, "Expand3 2":dbl}
  T15 = cluster{"Status":enum16{"Past", "Current", "Future"}, "x":dbl, "y":dbl, "z":dbl, "Vel":dbl, "Dwell Time":dbl, "BehCom":enum16{"Tug Off", "Manual Mode", "Goto WayPoint", "Back Up", "Gate", "Left Wall Follow", "Right Wall Follow", "Hunt"}, "Expand1":dbl, "Expand2":dbl, "Expand3":dbl, "Expand3 2":dbl}[]
  T16 = cluster{"Status":enum16{"Past", "Current", "Future"}, "x":dbl, "y":dbl, "z":dbl, "Vel":dbl, "Dwell Time":dbl, "BehCom":enum16{"Tug Off", "Manual Mode", "Goto WayPoint", "Back Up", "Gate", "Left Wall Follow", "Right Wall Follow", "Hunt"}, "X1":dbl, "Y1":dbl, "X2":dbl, "Y2":dbl}
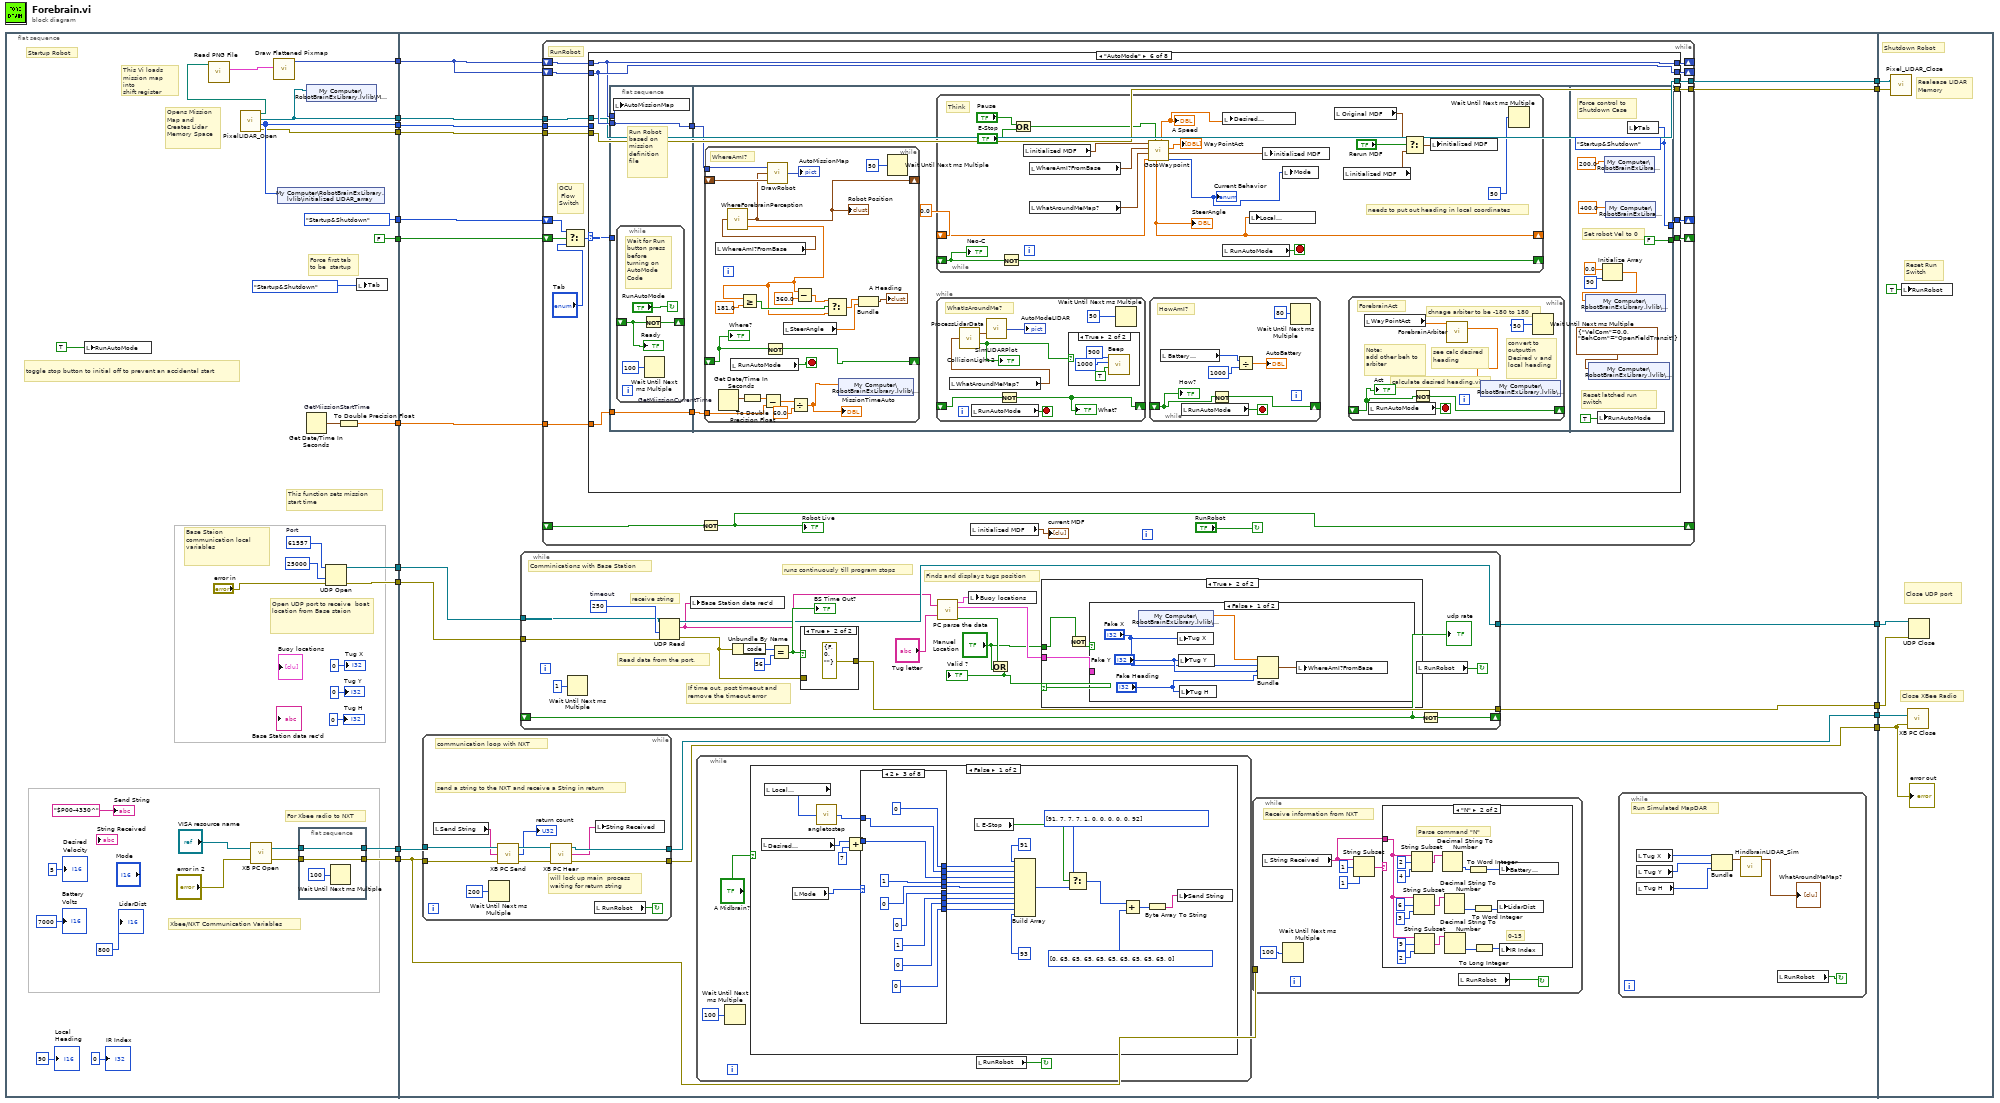
[diagram p0: block diagram]
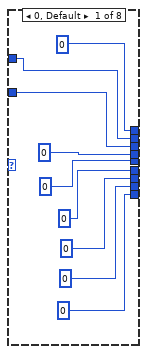
[diagram p2: hidden frame]
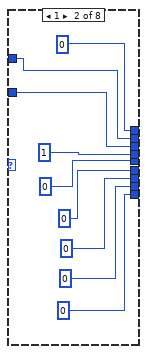
[diagram p3: hidden frame]
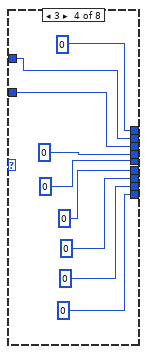
[diagram p4: hidden frame]
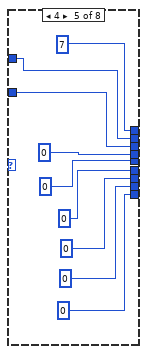
[diagram p5: hidden frame]
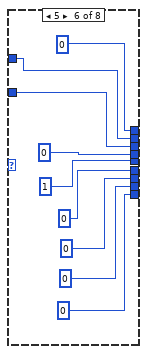
[diagram p6: hidden frame]
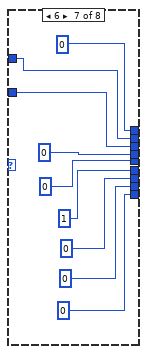
[diagram p7: hidden frame]
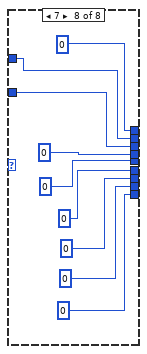
[diagram p8: hidden frame]
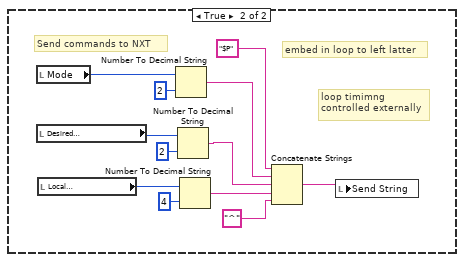
[diagram p9: hidden frame]
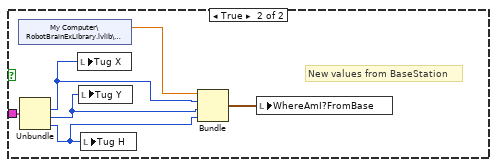
[diagram p12: hidden frame]
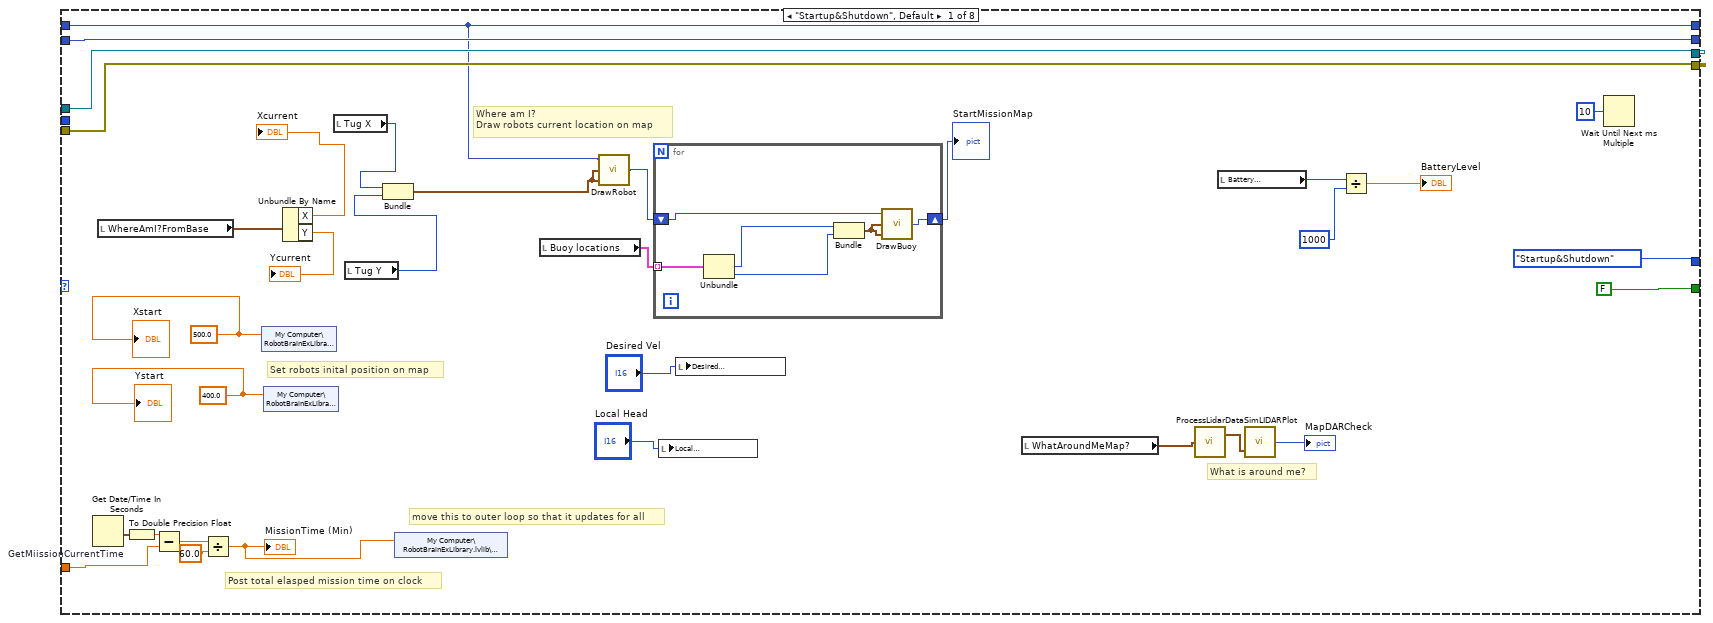
[diagram p14: hidden frame]
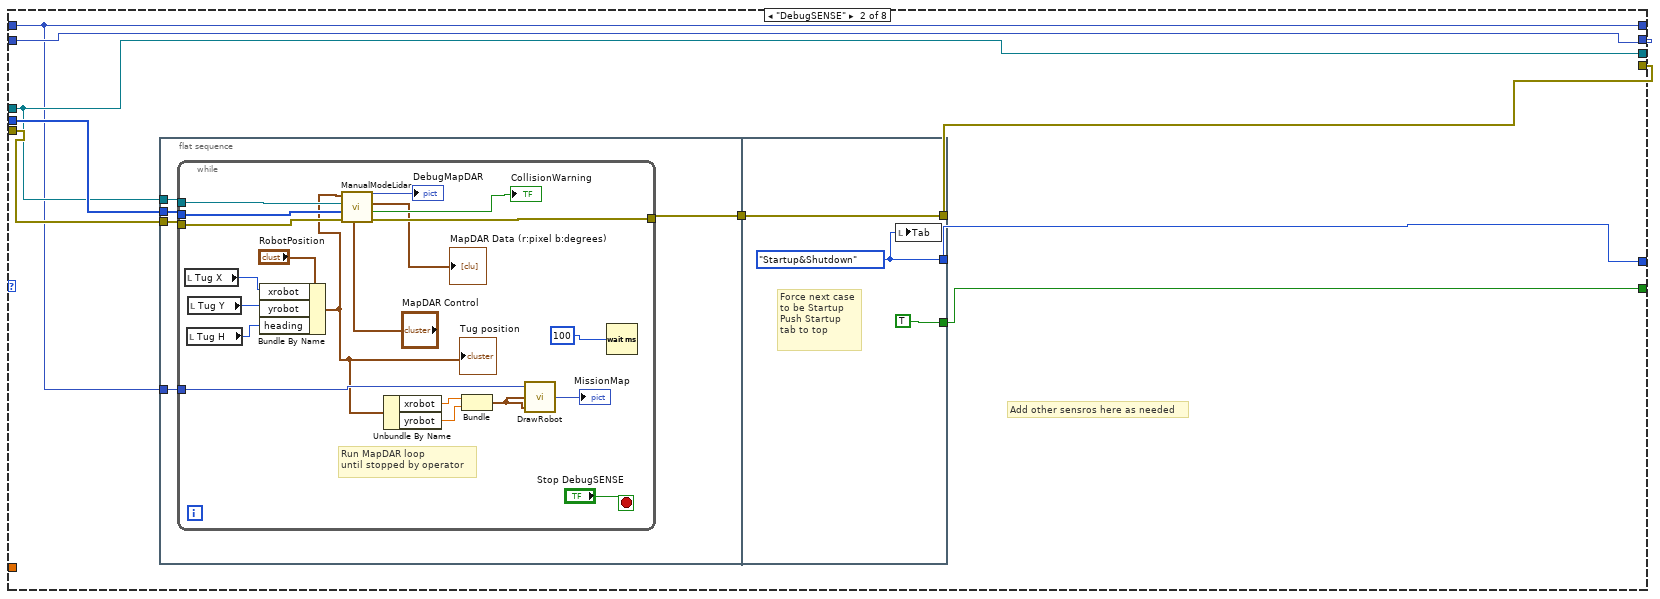
[diagram p15: hidden frame]
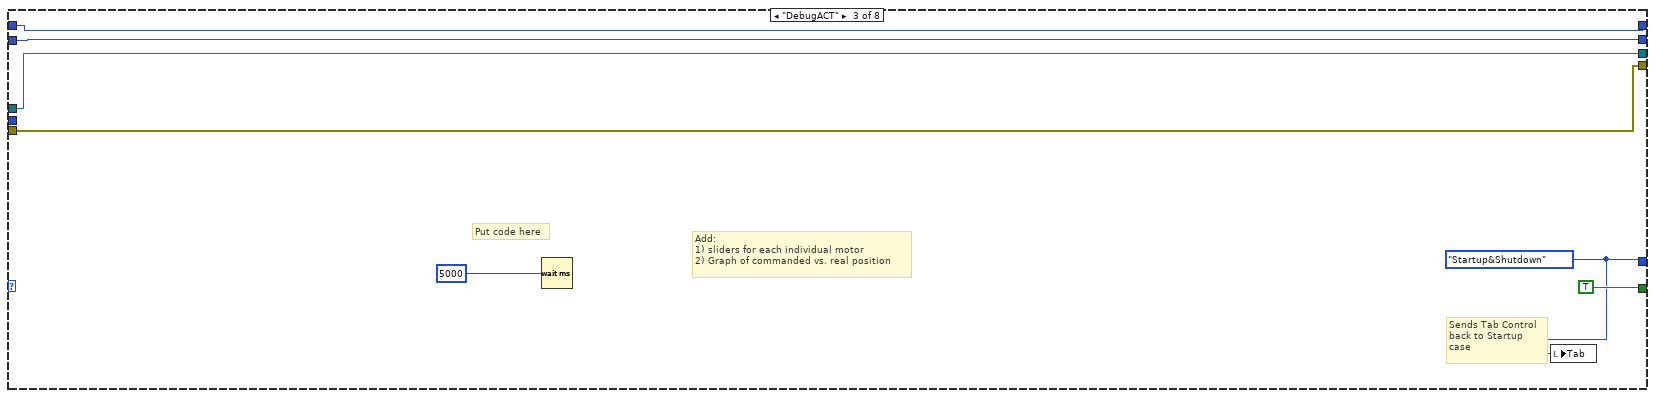
[diagram p16: hidden frame]
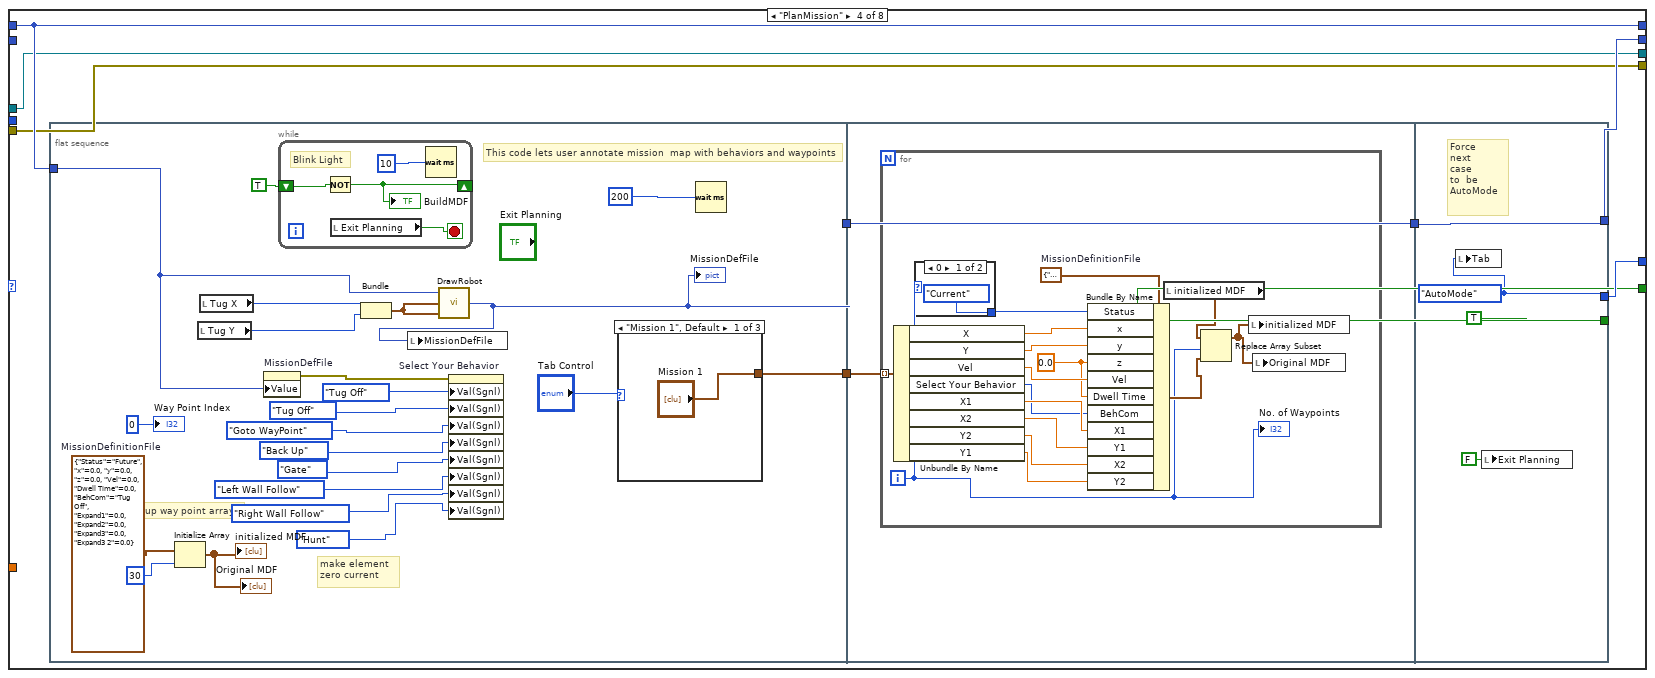
[diagram p17: hidden frame]
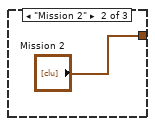
[diagram p18: hidden frame]
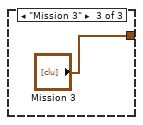
[diagram p19: hidden frame]
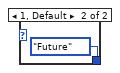
[diagram p20: hidden frame]
diagram:
  n1 = flat-sequence {
    tunnel: [w48] -> w17
    tunnel: [w47] -> w16
    tunnel: [w44] -> w15
    tunnel: [w46] -> w14
    tunnel: [w45] -> w13
    tunnel: [FALSE ("RunAutoMode")] -> w10
    tunnel: [T2."Startup&Shutdown" ("Tab")] -> w9
    tunnel: [w31] -> w8
    tunnel: [w30] -> w7
    tunnel: [w19] -> w6
    tunnel: [w18] -> w5
    tunnel: w17 -> [w69]
    tunnel: w16 -> [w68]
    tunnel: w15 -> [w67]
    tunnel: w14 -> [w66]
    tunnel: w13 -> [w65]
    tunnel: [w64] -> w12
    tunnel: [w63] -> w11
    tunnel: w10 -> [w62]
    tunnel: w9 -> [w61]
    tunnel: w8 -> [w56]
    tunnel: w7 -> [w55]
    tunnel: w6 -> [w60]
    tunnel: w5 -> [w57]
    tunnel: [w59] -> w4
    tunnel: [w58] -> w3
    tunnel: [w54] -> w2
    tunnel: [w53] -> w1
    tunnel: w12 -> [w608]
    tunnel: w11 -> [w607]
    tunnel: w4 -> [w606]
    tunnel: w3 -> [w605]
    tunnel: w2 -> [w604]
    tunnel: w1 -> [w603]
    frame #0 {
      w37 = u16 61557  # Port
      # "For Xbee radio to NXT"
      # "Xbee/NXT Communication Variables"
      # "Base Staion communication local variables"
      # "Open UDP port to receive  boat location from Base staion"
      # "Force first tab\nto be  startup"
      # "toggle stop button to initial off to prevent an accidental start"
      # "Opens Mission\nMap and\nCreates Lidar\nMemory Space"
      # "This function sets mission \nstart time"
      # "This Vi loads\nmission map into \nshift register"
      # "Startup Robot"
      n2 = local write "RunAutoMode"(TRUE ("RunAutoMode")) -> ()
      n3 = call "PixelLIDAR_Open.vi"() -> ("error out"=w45:errorcluster, "initialized LIDAR\narray"=w46:i32[], "MDF Image"=w44:T10, "MissionMap"=w39:path)  [unwired: 2 in]
      n4 = call <vilib>:"Read PNG File.vi"("path to PNG file"=w39) -> ("image data"=w38:T11)  [unwired: 8 in, 2 out]
      n5 = call "XB PC Open.vi"("error in (no error)"="error in 2", "VISA resource name"="VISA resource name") -> ("error out"=w22:errorcluster, "VISA resource name out"=w23:refnum<visa-resource-name>)
      n6 = call <vilib>:"Draw Flattened Pixmap.vi"("image data"=w38) -> ("new picture"=w47:picture)  [unwired: 8 in]
      n7 = shared-variable "My Computer\\RobotBrainExLibrary.lvlib\\initialized LIDAR_array"(w46) -> ()  [unwired: 1 in, 1 out]
      n8 = flat-sequence {
        tunnel: w23 -> [w50]
        tunnel: w22 -> [w51]
        tunnel: [w51] -> w18
        tunnel: [w50] -> w19
        frame #0 {
          n9 = Wait Until Next ms Multiple(millisecond multiple=u32 100) -> ()  [unwired: 1 out]
        }
      }
      n10 = shared-variable "My Computer\\RobotBrainExLibrary.lvlib\\MDF Image"(w44) -> ()  [unwired: 1 in, 1 out]
      n11 = Get Date/Time In Seconds "GetMiissionStartTime"() -> (seconds since 1Jan1904=w49:timestamp)
      n12 = UDP Open(8:"error in", 9:25000 ("timeout ms (25000)"), 11:w37) -> (port=w31:refnum<k16>, 0:w30:errorcluster)  [unwired: 2 in, 1 out]
      n13 = To Double Precision Float(number=w49) -> (double precision float=w48:dbl)
      n14 = local write "Tab"(T2."Startup&Shutdown" ("Tab")) -> ()
      "Tug X" <- 0 ("Tug X")
      "Tug Y" <- 0 ("Tug Y")
      "Tug H" <- 0 ("Tug H")
      "Battery\nVolts" <- i16 7000 ("Battery\nVolts")
      "LidarDist" <- i16 800 ("Dist")
      "IR Index" <- 0 ("IR Index")
      "Local\nHeading" <- i16 90 ("Local\nHeading")
      "Desired \nVelocity" <- i16 5 ("Desired \nVelocity")
      "Send String" <- "$P00-4330^"
    }
    frame #1 {
      n15 = while {
        tunnel: w60 -> [w219]
        tunnel: w57 -> [w218]
        tunnel: [w215] -> w58
        tunnel: [w214] -> w59
        stop <- w213 continue-if-true
        # "will lock up main  process\nwaiting for return string"
        # "communication loop with NXT"
        # "send a string to the NXT and receive a String in return"
        n16 = local read "Send String"() -> (w211:string)
        n17 = Wait Until Next ms Multiple(millisecond multiple=u32 200) -> ()  [unwired: 1 out]
        n18 = call "XB PC Send.vi"("error in (no error)"=w218, "String"=w211, "VISA resource name"=w219) -> ("error out"=w217:errorcluster, "return count"=→"return count":u32, "VISA resource name out"=w216:refnum<visa-resource-name>)
        n19 = call "XB PC Hear.vi"("VISA resource name"=w216, "error in (no error)"=w217) -> ("VISA resource name out"=w214:refnum<visa-resource-name>, "String Received"=w210:string, "error out"=w215:errorcluster)
        n20 = local read "RunRobot"() -> (w213:bool)
        n21 = local write "String Received"(w210) -> ()
      }
      n22 = while {
        tunnel: w56 -> [w232]
        tunnel: w55 -> [w231]
        tunnel: [w230] -> w53
        tunnel: [w229] -> w54
        shift-right: [w223] -> _
        shift-left: _ -> [w222]
        stop <- w233 continue-if-true
        w235 = 250  # timeout
        # "Finds and displays tugs position"
        # "runs continuously till program stops"
        # "Comminications with Base Station"
        # "receive string"
        # "If time out, post timeout and\nremove the timeout error"
        # "Read data from the port."
        n23 = Wait Until Next ms Multiple(millisecond multiple=u32 1) -> ()  [unwired: 1 out]
        n24 = UDP Read(connection ID=w232, timeout ms (25000)=w235, 8:w231) -> (data out=w224:string, error out=w236:errorcluster, 3:w229:refnum<k16>)  [unwired: 1 in, 2 out]
        n25 = local write "Base Station data rec'd"(w224) -> ()
        n26 = Unbundle By Name(w236) -> ("code"=w239:i32)
        n27 = Equal?(x=w239, y=56) -> (x = y?=w237:bool)
        "BS Time Out?" <- w237
        n28 = case shown="True" w237 {
          tunnel: [w254 errorcluster {"status"=FALSE, "code"=0, "source"=""} ("error out")] -> w230
          tunnel: w236 -> [w254 _]
          frame False {
          }
          frame True {
          }
        }
        n29 = call "PC parse the data.vi"("Nav String"=w224, "Tug"="Tug letter") -> ("Buoy locations"=w228:cluster{"regular expression":string, i32, i32}[], "Tug Location"=w226:T12, "Valid?"=w227:bool)  [unwired: 1 out]
        n30 = local write "Buoy locations"(w228) -> ()
        n31 = Or(x=w227, y="Manuel\nLocation") -> (x .or. y?=w221:bool)
        "Valid ?" <- w221
        n32 = case shown="True" w221 {
          tunnel: w226 -> [_ w242]
          tunnel: "Manuel\nLocation" -> [_ w240]
          frame False {
            # "No \nchange"
          }
          frame True {
            n33 = Not(x=w240) -> (.not. x?=w241:bool)
            n34 = case shown="False" w241 {
              tunnel: w242 -> [_ w253]
              frame False {
                n35 = shared-variable "My Computer\\RobotBrainExLibrary.lvlib\\MissionTime"() -> (w247:dbl)  [unwired: 1 in, 1 out]
                n36 = local write "Tug X"("Fake X") -> ()
                n37 = local write "Tug Y"("Fake Y") -> ()
                n38 = local write "Tug H"("Fake Heading") -> ()
                n39 = Bundle(w247, "Fake X"="Fake X", "Fake Y"="Fake Y", "Fake Heading"="Fake Heading") -> (w244:T13)  [unwired: 1 in]
                n40 = local write "WhereAmI?FromBase"(w244) -> ()
              }
              frame True {
                # "New values from BaseStation"
                n41 = shared-variable "My Computer\\RobotBrainExLibrary.lvlib\\MissionTime"() -> (w252:dbl)  [unwired: 1 in, 1 out]
                n42 = Unbundle(w253) -> (w251:i32, w250:i32, w249:i32)  [unwired: 1 out]
                n43 = local write "Tug X"(w251) -> ()
                n44 = local write "Tug Y"(w250) -> ()
                n45 = local write "Tug H"(w249) -> ()
                n46 = Bundle(w252, w251, w250, w249) -> (w248:cluster{dbl, i32, i32, i32})  [unwired: 1 in]
                n47 = local write "WhereAmI?FromBase"(w248) -> ()
              }
            }
          }
        }
        n48 = local read "RunRobot"() -> (w233:bool)
        n49 = Not(x=w222) -> (.not. x?=w223:bool)
        "udp rate" <- w222
      }
      n50 = while {
        shift-right: [w257] -> _
        shift-left: _ -> [w274]
        shift-right: [w273] -> _
        shift-left: w61 -> [w272]
        shift-right: [w269] -> _
        shift-left: w62 -> [w268]
        tunnel: w69 -> [w267]
        shift-right: [w265] -> _
        shift-left: w68 -> [w266]
        shift-right: [w263] -> _
        shift-left: w68 -> [w264]
        tunnel: w67 -> [w262]
        tunnel: w66 -> [w261]
        tunnel: w65 -> [w260]
        tunnel: [w259] -> w64
        tunnel: [w258] -> w63
        stop <- "RunRobot" continue-if-true
        # "RunRobot"
        # "OCU\n Flow\nSwitch"
        n51 = Select(t=w272, s=w268, f="Tab") -> (s? t:f=w270:T2)
        n52 = case shown="\"AutoMode\"" w270 {
          selector: w270 -> [_ _ _ _ _ w502 _ _]
          tunnel: [T2."Startup&Shutdown" ("Tab") w318 w355 w366 w426 w503 T2."Startup&Shutdown" ("Tab") w601] -> w273
          tunnel: [FALSE ("s") w317 TRUE ("s") w365 w427 w501 FALSE ("s") TRUE ("s")] -> w269
          tunnel: w267 -> [w301 _ _ _ w424 w499 _ _]
          tunnel: w266 -> [w277 w314 w354 w363 w422 w496 w592 w599]
          tunnel: [w277 w314 w354 w363 w422 w496 w592 w599] -> w265
          tunnel: w264 -> [w300 w315 w353 _ w423 w498 w591 w598]
          tunnel: [w300 w315 w353 w364 w423 w498 w591 w598] -> w263
          tunnel: w262 -> [w299 w316 w352 w359 w421 w495 w590 w597]
          tunnel: w261 -> [_ w322 _ _ _ _ _ _]
          tunnel: w260 -> [w298 w321 w351 w358 w420 w494 w589 w596]
          tunnel: [w299 w316 w352 w359 w421 w495 w590 w597] -> w259
          tunnel: [w298 w320 w351 w358 w420 w494 w589 w596] -> w258
          frame "Startup&Shutdown", Default {
            w291 = 400.0 ("Ystart")
            w292 = 500.0 ("Xstart")
            # "move this to outer loop so that it updates for all"
            # "Where am I?\nDraw robots current location on map"
            # "Post total elasped mission time on clock"
            # "What is around me?"
            # "Set robots inital position on map"
            n53 = Get Date/Time In Seconds "GetMiissionCurrentTime"() -> (seconds since 1Jan1904=w305:timestamp)
            n54 = local read "WhereAmI?FromBase"() -> (w281:T5)
            n55 = To Double Precision Float(number=w305) -> (double precision float=w304:dbl)
            n56 = Subtract(x=w304, y=w301) -> (x-y=w303:dbl)
            n57 = Divide(x=w303, y=60.0) -> (x/y=w297:dbl)
            "MissionTime (Min)" <- w297
            n58 = shared-variable "My Computer\\RobotBrainExLibrary.lvlib\\Xstart"(w292) -> ()  [unwired: 1 in, 1 out]
            n59 = shared-variable "My Computer\\RobotBrainExLibrary.lvlib\\Ystart"(w291) -> ()  [unwired: 1 in, 1 out]
            n60 = Unbundle By Name(w281) -> ("X"=→"Xcurrent":dbl, "Y"=→"Ycurrent":dbl)
            n61 = local read "Tug X"() -> (w290:i32)
            n62 = local read "Tug Y"() -> (w289:i32)
            n63 = Bundle("Tug X"=w290, "Tug Y"=w289) -> (w278:cluster{"Tug X":i32, "Tug Y":i32})  [unwired: 1 in]
            n64 = shared-variable "My Computer\\RobotBrainExLibrary.lvlib\\MissionTime"(w297) -> ()  [unwired: 1 in, 1 out]
            n65 = local read "Buoy locations"() -> (w280:cluster{"regular expression":string, i32, i32}[])
            n66 = call "DrawRobot.vi"("(xr,yr) old"=w278, "(xr,yr) new"=w278, "2D Picture"=w277) -> ("new picture"=w276:picture)
            n67 = for {
              shift-right: [w312] -> w279
              shift-left: w276 -> [w313]
              tunnel: w280 -> [w309] mode=indexing
              n68 = Unbundle(w309) -> (w311:i32, w310:i32)  [unwired: 1 out]
              n69 = Bundle(w311, w310) -> (w308:cluster{i32, i32})  [unwired: 1 in]
              n70 = call "DrawBuoy.vi"("(xr,yr) old"=w308, "(xr,yr) new"=w308, "2D Picture"=w313) -> ("new picture"=w312:picture)
            }
            "StartMissionMap" <- w279
            n71 = local write "Local\nHeading"("Local Head") -> ()
            n72 = local write "Desired \nVelocity"("Desired Vel") -> ()
            n73 = local read "WhatAroundMeMap?"() -> (w282:cluster{"T":dbl, "Range":dbl, "Bearing":dbl}[])
            n74 = call "ProcessLidarData.vi"("WhatAroundMe?MM"=w282) -> ("data array [mag, phase (deg)]"=w295:cluster{"magnitude":dbl, "phase":dbl}[])  [unwired: 1 out]
            n75 = local read "Battery\nVolts"() -> (w286:i16)
            n76 = call "SimLIDARPlot.vi"("data array [mag, phase (deg)]"=w295) -> ("SONAR"=→"MapDARCheck":picture)  [unwired: 1 in]
            n77 = Divide(x=w286, y=i16 1000) -> (x/y=→"BatteryLevel":dbl)
            n78 = Wait Until Next ms Multiple(millisecond multiple=u32 10) -> ()  [unwired: 1 out]
            "Xstart" <- w292
            "Ystart" <- w291
          }
          frame "DebugSENSE" {
            # "Add other sensros here as needed"
            n79 = flat-sequence {
              tunnel: w322 -> [w327]
              tunnel: w321 -> [w326]
              tunnel: w316 -> [w325]
              tunnel: [w324] -> w319
              tunnel: w314 -> [w323]
              tunnel: [w350] -> w320
              tunnel: w319 -> [w350]
              tunnel: [w349] -> w318
              tunnel: [TRUE ("s")] -> w317
              frame #0 {
                n80 = while {
                  tunnel: w327 -> [w347]
                  tunnel: w326 -> [w346]
                  tunnel: w325 -> [w345]
                  tunnel: [w344] -> w324
                  tunnel: w323 -> [w338]
                  stop <- "Stop DebugSENSE" stop-if-true
                  # "Run MapDAR loop\nuntil stopped by operator"
                  n81 = local read "Tug X"() -> (w332:i32)
                  n82 = local read "Tug H"() -> (w333:i32)
                  n83 = local read "Tug Y"() -> (w331:i32)
                  n84 = Bundle By Name(cluster="RobotPosition", "xrobot"=w332, "yrobot"=w331, "heading"=w333) -> (w329:T4)
                  "Tug position" <- w329
                  n85 = call "ManualModeLidar.vi"("LIDARControl"="MapDAR Control", "error in"=w346, "initialized \nsonar ray\narray"=w347, "MDF Image"=w345, "SubPosition"=w329) -> ("error out"=w344:errorcluster, "Collision\nWarning"=→"CollisionWarning":bool, "LIDAR Data (r:pixel b:degrees)"=→"MapDAR Data (r:pixel b:degrees)":cluster{"Range":dbl, "Bearing":dbl}[], "LIDAR"=→"DebugMapDAR":picture)  [unwired: 1 in]
                  n86 = Unbundle By Name(w329) -> ("xrobot"=w336:dbl, "yrobot"=w335:dbl)
                  n87 = Bundle("xrobot"=w336, "yrobot"=w335) -> (w328:cluster{"xrobot":dbl, "yrobot":dbl})  [unwired: 1 in]
                  n88 = call "DrawRobot.vi"("(xr,yr) old"=w328, "(xr,yr) new"=w328, "2D Picture"=w338) -> ("new picture"=→"MissionMap":picture)
                  n89 = Wait (ms)(milliseconds to wait=u32 100) -> ()  [unwired: 1 out]
                }
              }
              frame #1 {
                w349 = T2."Startup&Shutdown" ("Tab")
                # "Force next case\nto be Startup\nPush Startup\ntab to top"
                n90 = local write "Tab"(w349) -> ()
              }
            }
          }
          frame "DebugACT" {
            w355 = T2."Startup&Shutdown" ("Tab")
            # "Add:\n1) sliders for each individual motor\n2) Graph of commanded vs. real position"
            # "Put code here"
            # "Sends Tab Control\nback to Startup\ncase"
            n91 = Wait (ms)(milliseconds to wait=u32 5000) -> ()  [unwired: 1 out]
            n92 = local write "Tab"(w355) -> ()
          }
          frame "PlanMission" {
            n93 = flat-sequence {
              tunnel: [w376] -> w362
              tunnel: w363 -> [w382]
              tunnel: [w377] -> w360
              tunnel: w362 -> [w397]
              tunnel: [w397] -> w361
              tunnel: w360 -> [w396]
              tunnel: [w418] -> w366
              tunnel: [TRUE ("s")] -> w365
              tunnel: w361 -> [w417]
              tunnel: [w417] -> w364
              frame #0 {
                w381 = T14 {"Status"=enum."Future", "x"=0.0, "y"=0.0, "z"=0.0, "Vel"=0.0, "Dwell Time"=0.0, "BehCom"=enum."Tug Off", "Expand1"=0.0, "Expand2"=0.0, "Expand3"=0.0, "Expand3 2"=0.0}  # MissionDefinitionFile
                # "make element \nzero current"
                # "sets up way point array"
                # "This code lets user annotate mission  map with behaviors and waypoints"
                n94 = Initialize Array ("Initialize WaypointArray")(w381, 30 ("dimension size")) -> (→"initialized MDF" →"Original MDF":T15)
                n95 = local read "Tug Y"() -> (w379:i32)
                n96 = local read "Tug X"() -> (w380:i32)
                n97 = property on="MissionDefFile" class="Pict"("Value"=w382) -> (error out=w387:errorcluster)  [unwired: 2 in, 1 out]
                n98 = while {
                  shift-right: [w394] -> _
                  shift-left: TRUE -> [w395]
                  stop <- w393 stop-if-true
                  # "Blink Light"
                  n99 = Not(x=w395) -> (.not. x?=w394:bool)
                  "BuildMDF" <- w394
                  n100 = local read "Exit Planning"() -> (w393:bool)
                  n101 = Wait (ms)(milliseconds to wait=u32 10) -> ()  [unwired: 1 out]
                }
                n102 = Bundle("Tug X"=w380, "Tug Y"=w379) -> (w383:cluster{"Tug X":i32, "Tug Y":i32})  [unwired: 1 in]
                n103 = call "DrawRobot.vi"("(xr,yr) old"=w383, "(xr,yr) new"=w383, "2D Picture"=w382) -> ("new picture"=w376:picture)
                "MissionDefFile" <- w376
                n104 = local write "MissionDefFile"(w376) -> ()
                n105 = property on="Select Your Behavior" class="Enum (strict)"(error in=w387, "Val(Sgnl)"=T8."Tug Off" ("Value (Signaling)"), "Val(Sgnl)"=T8."Tug Off" ("Value (Signaling)"), "Val(Sgnl)"=T8."Goto WayPoint" ("Value (Signaling)"), "Val(Sgnl)"=T8."Back Up" ("Value (Signaling)"), "Val(Sgnl)"=T8."Gate" ("Value (Signaling)"), "Val(Sgnl)"=T8."Left Wall Follow" ("Value (Signaling)"), "Val(Sgnl)"=T8."Right Wall Follow" ("Value (Signaling)"), "Val(Sgnl)"=T8."Hunt" ("Value (Signaling)")) -> ()  [unwired: 1 in, 2 out]
                n106 = case shown="\"Mission 1\", Default" "Tab Control" {
                  tunnel: ["Mission 1" "Mission 2" "Mission 3"] -> w377
                  frame "Mission 1", Default {
                  }
                  frame "Mission 2" {
                  }
                  frame "Mission 3" {
                  }
                }
                n107 = Wait (ms)(milliseconds to wait=u32 200) -> ()  [unwired: 1 out]
                "Way Point Index" <- 0 ("Boundary Point Index")
              }
              frame #1 {
                n108 = for {
                  tunnel: w396 -> [w413] mode=indexing
                  i -> [w403]
                  w411 = T16 {"Status"=enum."Future", "x"=0.0, "y"=0.0, "z"=0.0, "Vel"=0.0, "Dwell Time"=0.0, "BehCom"=enum."Tug Off", "X1"=0.0, "Y1"=0.0, "X2"=0.0, "Y2"=0.0}  # MissionDefinitionFile
                  w406 = 0.0 ("z")
                  n109 = Unbundle By Name(w413) -> ("X"=w409:dbl, "Y"=w408:dbl, "Vel"=w407:dbl, "Select Your Behavior"=w398:T8, "X1"=w402:dbl, "X2"=w401:dbl, "Y2"=w400:dbl, "Y1"=w399:dbl)
                  n110 = case shown="0" w403 {
                    tunnel: [enum16{"Past", "Current", "Future"}."Current" enum16{"Past", "Current", "Future"}."Future"] -> w405
                    frame 0 {
                    }
                    frame 1, Default {
                    }
                  }
                  n111 = Bundle By Name(cluster=w411, "Status"=w405, "x"=w409, "y"=w408, "z"=w406, "Vel"=w407, "Dwell Time"=w406, "BehCom"=w398, "X1"=w402, "Y1"=w401, "X2"=w400, "Y2"=w399) -> (w410:T16)
                  n112 = local read "initialized MDF"() -> (w412:T1)
                  n113 = Replace Array Subset(array=w412, new element=w410, index=w403) -> (w404:T1)
                  n114 = local write "initialized MDF"(w404) -> ()
                  n115 = local write "Original MDF"(w404) -> ()
                  "No. of Waypoints" <- w403
                }
              }
              frame #2 {
                w418 = T2."AutoMode" ("Tab")
                # "Force \nnext \ncase\nto  be\nAutoMode"
                n116 = local write "Tab"(w418) -> ()
                n117 = local write "Exit Planning"(FALSE ("Exit Planning")) -> ()
              }
            }
          }
          frame "ManualMode" {
            # "Removing map shift register\nfixed memory leak?"
            # "Manual Steering by dashboard heading steering wheel\nand by speed slider"
            # "This mode lets \noperator directly\ndrive robot via\nthe ManualMode\ntabbed interface"
            n118 = while {
              shift-right: [w450] -> _
              shift-left: _ -> [w449]
              tunnel: w424 -> [w442]
              shift-right: [w439] -> _
              shift-left: _ -> [w438]
              tunnel: w422 -> [w436]
              stop <- w448 stop-if-true
              # "WhereAmI?"
              n119 = Get Date/Time In Seconds "GetMiissionCurrentTime"() -> (seconds since 1Jan1904=w443:timestamp)
              n120 = call "WhereForebrainPerception.vi"("Where? Midbrain"="WhereAmI?FromBase") -> ("Where? Forebrain"=→"Where? Manual":T5, "(xr,yr)"=w439:cluster{"X":dbl, "Y":dbl}, "Direction"=w428:dbl)  [unwired: 3 in, 1 out]
              "(xr,yr)" <- w439
              n121 = local read "ManualModeStop"() -> (w448:bool)
              n122 = To Double Precision Float(number=w443) -> (double precision float=w444:dbl)
              n123 = Greater Or Equal?(x=w428, y=181.0) -> (x >= y?=w433:bool)
              n124 = local read "Manual Heading"() -> (w440:i16)
              n125 = Subtract(x=w444, y=w442) -> (x-y=w445:dbl)
              n126 = Not(x=w449) -> (.not. x?=w450:bool)
              n127 = call "DrawRobot.vi"("(xr,yr) old"=w438, "(xr,yr) new"=w439, "2D Picture"=w436) -> ("new picture"=→"ManualMissionMap":picture)
              n128 = Divide(x=w445, y=60.0) -> (x/y=w447:dbl)
              "MissionTime" <- w447
              n129 = Subtract(x=w428, y=360.0) -> (x-y=w431:dbl)
              n130 = shared-variable "My Computer\\RobotBrainExLibrary.lvlib\\MissionTime"(w447) -> ()  [unwired: 1 in, 1 out]
              n131 = Select(t=w431, s=w433, f=w428) -> (s? t:f=w430:dbl)
              n132 = Bundle("Direction"=w430, "Manual Heading"=w440) -> (→"Heading":cluster{"Direction":dbl, "Manual Heading":i16})  [unwired: 1 in]
              n133 = Wait Until Next ms Multiple(millisecond multiple=u32 100 ("milliseconds to wait")) -> ()  [unwired: 1 out]
              "Where? 2" <- w449
            }
            n134 = while {
              shift-right: [w457] -> _
              shift-left: _ -> [w458]
              stop <- "ManualModeStop" stop-if-true
              # "WhatIsAroundMe?"
              n135 = local read "WhatAroundMeMap?"() -> (w452:cluster{"T":dbl, "Range":dbl, "Bearing":dbl}[])
              n136 = call "ProcessLidarData.vi"("WhatAroundMe?MM"=w452) -> ("Collision"=w453:bool, "data array [mag, phase (deg)]"=w454:cluster{"magnitude":dbl, "phase":dbl}[])
              "CollisionLight" <- w453
              n137 = Not(x=w458) -> (.not. x?=w457:bool)
              "MWhat?" <- w457
              n138 = call "SimLIDARPlot.vi"("data array [mag, phase (deg)]"=w454) -> ("SONAR"=→"ManualModeMapDAR":picture)  [unwired: 1 in]
              n139 = case shown="True" w453 {
                frame False {
                  # "No \nBeep"
                }
                frame True {
                  n140 = call <vilib>:"Beep.vi"("use system alert? (T)"=TRUE, "duration (msec)"=u32 1000, "frequency (Hz)"=u32 900) -> ()  [unwired: 9 in]
                }
              }
              n141 = Wait Until Next ms Multiple(millisecond multiple=u32 100 ("milliseconds to wait")) -> ()  [unwired: 1 out]
            }
            n142 = while {
              shift-right: [w481] -> _
              shift-left: _ -> [w480]
              stop <- w479 stop-if-true
              # "HowAmI?"
              n143 = local read "Battery\nVolts"() -> (w478:i16)
              n144 = local read "ManualModeStop"() -> (w479:bool)
              n145 = Not(x=w480) -> (.not. x?=w481:bool)
              n146 = Divide(x=w478, y=i16 1000) -> (x/y=→"Battery":dbl)
              n147 = Wait Until Next ms Multiple(millisecond multiple=u32 100 ("milliseconds to wait")) -> ()  [unwired: 1 out]
              "How? 2" <- w480
            }
            n148 = while {
              shift-right: [w475] -> _
              shift-left: _ -> [w474]
              stop <- w473 stop-if-true
              # "ForebrainAct"
              n149 = local read "E-Stop"() -> (w471:bool)
              n150 = local read "ManualModeStop"() -> (w473:bool)
              n151 = Select(t=0.0, s=w471, f="Manual Vel") -> (s? t:f=w468:dbl)
              n152 = To Word Integer(number=w468) -> (16bit integer=w466:i16)
              "Speed" <- w466
              n153 = local read "Send String"() -> (→"Send String to NXT":string)
              n154 = To Word Integer(number="Behavior Command") -> (16bit integer=w463:i16)
              n155 = local write "Mode"(w463) -> ()
              n156 = local write "Desired \nVelocity"(w466) -> ()
              n157 = local write "Local\nHeading"("Manual Heading") -> ()
              n158 = Not(x=w474) -> (.not. x?=w475:bool)
              n159 = Wait Until Next ms Multiple(millisecond multiple=u32 50 ("milliseconds to wait")) -> ()  [unwired: 1 out]
              "ActManual" <- w474
            }
            n160 = local read "ManualModeStop"() -> (w425:bool)
            n161 = case shown="True" w425 {
              tunnel: [TRUE ("s") w485] -> w427
              tunnel: [T2."ManualMode" ("Tab") w486] -> w426
              frame False {
              }
              frame True {
                # "Debounce tab for clean transition"
                n162 = flat-sequence {
                  tunnel: [w492] -> w486
                  tunnel: [TRUE ("s")] -> w485
                  frame #0 {
                    n163 = Wait (ms)(milliseconds to wait=u32 100) -> ()  [unwired: 1 out]
                  }
                  frame #1 {
                    w492 = T2."Startup&Shutdown" ("Tab")
                    # "Turn off\nVelocity\non \nExit"
                    n164 = local write "ManualModeStop"(FALSE ("ManualModeStop")) -> ()
                    n165 = local write "Desired \nVelocity"(i16 0 ("Desired \nVelocity")) -> ()
                    n166 = local write "Local\nHeading"(i16 0 ("Local\nHeading")) -> ()
                    n167 = local write "Mode"(i16 0 ("Mode")) -> ()
                    n168 = local write "Tab"(w492) -> ()
                  }
                }
              }
            }
          }
          frame "AutoMode" {
            n169 = flat-sequence {
              tunnel: w502 -> [_]
              tunnel: [w505] -> w500
              tunnel: w499 -> [w505]
              tunnel: w498 -> [w504]
              tunnel: [w504] -> w497
              tunnel: w496 -> [_]
              tunnel: w500 -> [w512]
              tunnel: w497 -> [w510]
              tunnel: [w587] -> w503
              tunnel: [FALSE ("s")] -> w501
              frame #0 {
                # "Run Robot\nbased on\nmission\ndefinition\nfile"
                n170 = local write "AutoMissionMap"(w504) -> ()
                n171 = while {
                  shift-right: [w508] -> _
                  shift-left: _ -> [w507]
                  stop <- "RunAutoMode" continue-if-true
                  # "Wait for Run\nbutton press\nbefore\nturning on\nAutoMode\nCode"
                  n172 = Not(x=w507) -> (.not. x?=w508:bool)
                  n173 = Wait Until Next ms Multiple(millisecond multiple=u32 100 ("milliseconds to wait")) -> ()  [unwired: 1 out]
                  "Ready" <- w507
                }
              }
              frame #1 {
                n174 = while {
                  shift-right: [w558] -> _
                  shift-left: _ -> [w549]
                  tunnel: w512 -> [w553]
                  shift-right: [w551] -> _
                  shift-left: _ -> [w552]
                  tunnel: w510 -> [w544]
                  stop <- w548 stop-if-true
                  # "WhereAmI?"
                  n175 = local read "WhereAmI?FromBase"() -> (w543:T5)
                  n176 = Get Date/Time In Seconds "GetMiissionCurrentTime"() -> (seconds since 1Jan1904=w554:timestamp)
                  n177 = call "WhereForebrainPerception.vi"("Where? Midbrain"=w543) -> ("(xr,yr)"=w551:cluster{"X":dbl, "Y":dbl}, "Direction"=w537:dbl)  [unwired: 3 in, 2 out]
                  "Robot Position" <- w551
                  n178 = local read "RunAutoMode"() -> (w548:bool)
                  n179 = Greater Or Equal?(x=w537, y=181.0) -> (x >= y?=w541:bool)
                  n180 = To Double Precision Float(number=w554) -> (double precision float=w555:dbl)
                  n181 = Subtract(x=w555, y=w553) -> (x-y=w556:dbl)
                  n182 = Not(x=w549) -> (.not. x?=w558:bool)
                  n183 = call "DrawRobot.vi"("(xr,yr) old"=w552, "(xr,yr) new"=w551, "2D Picture"=w544) -> ("new picture"=→"AutoMissionMap":picture)
                  n184 = local read "SteerAngle"() -> (w546:dbl)
                  n185 = Divide(x=w556, y=60.0) -> (x/y=w550:dbl)
                  "MissionTimeAuto" <- w550
                  n186 = Subtract(x=w537, y=360.0) -> (x-y=w539:dbl)
                  n187 = Select(t=w539, s=w541, f=w537) -> (s? t:f=w538:dbl)
                  n188 = shared-variable "My Computer\\RobotBrainExLibrary.lvlib\\MissionTime"(w550) -> ()  [unwired: 1 in, 1 out]
                  n189 = Bundle("Direction"=w538, "SteerAngle"=w546) -> (→"A Heading":cluster{"Direction":dbl, "SteerAngle":dbl})  [unwired: 1 in]
                  n190 = Wait Until Next ms Multiple(millisecond multiple=u32 50 ("milliseconds to wait")) -> ()  [unwired: 1 out]
                  "Where?" <- w549
                }
                n191 = while {
                  shift-right: [w577] -> _
                  shift-left: _ -> [w576]
                  shift-right: [w567] -> _
                  shift-left: 0.0 ("SteerAngle") -> [w572]
                  stop <- w579 stop-if-true
                  # "needs to put out heading in local coordinates"
                  # "Think"
                  n192 = Not(x=w576) -> (.not. x?=w577:bool)
                  n193 = Or(x="Pause", y="E-Stop") -> (x .or. y?=w569:bool)
                  n194 = local read "initialized MDF"() -> (w561:T1)
                  n195 = local read "WhereAmI?FromBase"() -> (w575:T5)
                  n196 = local read "WhatAroundMeMap?"() -> (w574:cluster{"T":dbl, "Range":dbl, "Bearing":dbl}[])
                  n197 = call "GotoWaypoint.vi"("InhibitIn"=w569, "CurrentSteerAngle"=w572, "WhatAroundMe? Clean"=w574, "WhereAmI? Clean"=w575, "MDF In"=w561) -> ("BehCom"=w562:T7, "MDF Out"=w560:T1, "ActCommand"=→"WayPointAct":dbl[], "Vel"=w566:dbl, "SteerAngle"=w567:dbl)  [unwired: 1 in, 1 out]
                  "SteerAngle" <- w567
                  "A Speed" <- w566
                  "Current Behavior" <- w562
                  n198 = local write "Desired \nVelocity"(w566) -> ()
                  n199 = local read "RunAutoMode"() -> (w579:bool)
                  n200 = local write "Local\nHeading"(w567) -> ()
                  n201 = local write "initialized MDF"(w560) -> ()
                  n202 = local write "Mode"(w562) -> ()
                  n203 = local read "Original MDF"() -> (w565:T1)
                  n204 = local read "initialized MDF"() -> (w564:T1)
                  n205 = Select(t=w565, s="Rerun MDF", f=w564) -> (s? t:f=w563:T1)
                  n206 = local write "initialized MDF"(w563) -> ()
                  n207 = Wait Until Next ms Multiple(millisecond multiple=u32 50 ("milliseconds to wait")) -> ()  [unwired: 1 out]
                  "Neo-C" <- w576
                }
                n208 = while {
                  shift-right: [w530] -> _
                  shift-left: _ -> [w532]
                  stop <- w529 stop-if-true
                  # "WhatIsAroundMe?"
                  n209 = local read "WhatAroundMeMap?"() -> (w526:cluster{"T":dbl, "Range":dbl, "Bearing":dbl}[])
                  n210 = call "ProcessLidarData.vi"("WhatAroundMe?MM"=w526) -> ("Collision"=w527:bool, "data array [mag, phase (deg)]"=w531:cluster{"magnitude":dbl, "phase":dbl}[])
                  "CollisionLight 2" <- w527
                  n211 = local read "RunAutoMode"() -> (w529:bool)
                  n212 = call "SimLIDARPlot.vi"("data array [mag, phase (deg)]"=w531) -> ("SONAR"=→"AutoModeLIDAR":picture)  [unwired: 1 in]
                  n213 = Not(x=w532) -> (.not. x?=w530:bool)
                  "What?" <- w530
                  n214 = case shown="True" w527 {
                    frame False {
                      # "No \nBeep"
                    }
                    frame True {
                      n215 = call <vilib>:"Beep.vi"("use system alert? (T)"=TRUE, "duration (msec)"=u32 1000, "frequency (Hz)"=u32 900) -> ()  [unwired: 9 in]
                    }
                  }
                  n216 = Wait Until Next ms Multiple(millisecond multiple=u32 50 ("milliseconds to wait")) -> ()  [unwired: 1 out]
                }
                n217 = while {
                  shift-right: [w524] -> _
                  shift-left: _ -> [w523]
                  stop <- w522 stop-if-true
                  # "HowAmI?"
                  n218 = local read "Battery\nVolts"() -> (w520:i16)
                  n219 = local read "RunAutoMode"() -> (w522:bool)
                  n220 = Not(x=w523) -> (.not. x?=w524:bool)
                  n221 = Divide(x=w520, y=i16 1000) -> (x/y=→"AutoBattery":dbl)
                  n222 = Wait Until Next ms Multiple(millisecond multiple=u32 80 ("milliseconds to wait")) -> ()  [unwired: 1 out]
                  "How?" <- w523
                }
                n223 = while {
                  shift-right: [w517] -> _
                  shift-left: _ -> [w516]
                  stop <- w515 stop-if-true
                  # "calculate desired heading.vi"
                  # "see calc desired\nheading"
                  # "convert to \noutputtin\nDesired v and\nlocal heading"
                  # "chnage arbiter to be -180 to 180"
                  # "Note:\nadd other beh to\narbiter"
                  # "ForebrainAct"
                  n224 = local read "WayPointAct"() -> (w514:dbl[])
                  n225 = local read "RunAutoMode"() -> (w515:bool)
                  n226 = Not(x=w516) -> (.not. x?=w517:bool)
                  n227 = call "ForebrainArbiter.vi"("WaypointInput"=w514) -> ("ForebrainActCom"=w513:dbl[])  [unwired: 14 in]
                  n228 = shared-variable "My Computer\\RobotBrainExLibrary.lvlib\\ActCommand"(w513) -> ()  [unwired: 1 in, 1 out]
                  n229 = Wait Until Next ms Multiple(millisecond multiple=u32 50 ("milliseconds to wait")) -> ()  [unwired: 1 out]
                  "Act" <- w516
                }
              }
              frame #2 {
                w587 = T2."Startup&Shutdown" ("Tab")
                # "Set robot Vel to 0"
                # "Reset latched run\nswitch"
                # "Force control to\nShutdown Case"
                n230 = shared-variable "My Computer\\RobotBrainExLibrary.lvlib\\ForebrainCom"(T9 {"VelCom"=0.0, "BehCom"=enum."OpenFieldTransit"} ("ForebrainCom")) -> ()  [unwired: 1 in, 1 out]
                n231 = local write "RunAutoMode"(TRUE ("RunAutoMode")) -> ()
                n232 = Initialize Array(0.0 ("element"), 90 ("dimension size")) -> (w583:dbl[])
                n233 = shared-variable "My Computer\\RobotBrainExLibrary.lvlib\\ActCommand"(w583) -> ()  [unwired: 1 in, 1 out]
                n234 = shared-variable "My Computer\\RobotBrainExLibrary.lvlib\\Xstart"(200.0 ("Xstart")) -> ()  [unwired: 1 in, 1 out]
                n235 = shared-variable "My Computer\\RobotBrainExLibrary.lvlib\\Ystart"(400.0 ("Ystart")) -> ()  [unwired: 1 in, 1 out]
                n236 = local write "Tab"(w587) -> ()
              }
            }
          }
          frame "Documentation" {
            # "Add:\n1) Blinking lights in each loop to show that they are running"
            # "This mode is just a static data flow picture of the ForeBrain"
            n237 = Wait (ms)(milliseconds to wait=u32 500) -> ()  [unwired: 1 out]
          }
          frame "DebugTHINK" {
            w601 = T2."Startup&Shutdown" ("Tab")
            # "Add:\n1) a button for each midbrain behavior to help in debugging\n2) graph of \"neural\" arbiter brain waves for each actuator\n3) a button for each forebrain behavior"
            # "Put code here in place of delay"
            # "Sends Tab Control\nback to Startup\ncase"
            n238 = Wait (ms)(milliseconds to wait=u32 5000) -> ()  [unwired: 1 out]
            n239 = local write "Tab"(w601) -> ()
          }
        }
        n240 = Not(x=w274) -> (.not. x?=w257:bool)
        "Robot Live" <- w257
        n241 = local read "initialized MDF"() -> (→"current MDF":T1)
      }
      n242 = while {
        stop <- w72 continue-if-true
        n243 = Wait Until Next ms Multiple(millisecond multiple=u32 100) -> ()  [unwired: 1 out]
        n244 = case shown="False" "A Midbrain?" {
          frame False {
            n245 = local read "Desired \nVelocity"() -> (w76:i16)
            n246 = local read "Local\nHeading"() -> (w78:i16)
            n247 = local read "Mode"() -> (w73:i16)
            n248 = call "angletostep.vi"("Angle"=w78) -> ("Step"=w77:i16)
            n249 = Add(x=w76, y=7) -> (x+y=w75:i32)
            n250 = case shown="2" w73 {
              tunnel: [w103 w112 w121 w130 w139 w148 w157 w166] -> w96
              tunnel: [w104 w113 w122 w131 w140 w149 w158 w167] -> w95
              tunnel: [u8 0 ("# 6") u8 0 ("# 6") u8 0 ("# 6") u8 0 ("# 6") u8 0 ("# 6") u8 0 ("# 6") u8 0 ("# 6") u8 0 ("# 6")] -> w87
              tunnel: [u8 0 ("# 6") u8 0 ("# 6") u8 0 ("# 6") u8 0 ("# 6") u8 0 ("# 6") u8 0 ("# 6") u8 0 ("# 6") u8 0 ("# 6")] -> w86
              tunnel: [u8 0 ("# 6") u8 0 ("# 6") u8 1 ("# 6") u8 0 ("# 6") u8 0 ("# 6") u8 0 ("# 6") u8 0 ("# 6") u8 0 ("# 6")] -> w85
              tunnel: [u8 0 ("# 6") u8 0 ("# 6") u8 0 ("# 6") u8 0 ("# 6") u8 0 ("# 6") u8 0 ("# 6") u8 1 ("# 6") u8 0 ("# 6")] -> w84
              tunnel: [u8 0 ("# 6") u8 0 ("# 6") u8 0 ("# 6") u8 0 ("# 6") u8 0 ("# 6") u8 1 ("# 6") u8 0 ("# 6") u8 0 ("# 6")] -> w83
              tunnel: [u8 0 ("# 6") u8 1 ("# 6") u8 1 ("# 6") u8 0 ("# 6") u8 0 ("# 6") u8 0 ("# 6") u8 0 ("# 6") u8 0 ("# 6")] -> w82
              tunnel: [u8 0 ("IR Servo") u8 0 ("IR Servo") u8 0 ("IR Servo") u8 0 ("IR Servo") u8 7 ("IR Servo") u8 0 ("IR Servo") u8 0 ("IR Servo") u8 0 ("IR Servo")] -> w81
              tunnel: w77 -> [w104 w113 w122 w131 w140 w149 w158 w167]
              tunnel: w75 -> [w103 w112 w121 w130 w139 w148 w157 w166]
              frame 0, Default {
              }
              frame 1 {
              }
              frame 2 {
              }
              frame 3 {
              }
              frame 4 {
              }
              frame 5 {
              }
              frame 6 {
              }
              frame 7 {
              }
            }
            n251 = local read "E-Stop"() -> (w79:bool)
            n252 = Build Array(u8 91 ("element"), w81, w95, w96, w82, w83, w84, w85, w86, w87, u8 93 ("element")) -> (w88:i32[])
            n253 = Select(t=u8[] [91, 7, 7, 7, 1, 0, 0, 0, 0, 0, 92], s=w79, f=w88) -> (s? t:f=w89:i32[])
            n254 = Add(x=w89, y=u8[] [0, 65, 65, 65, 65, 65, 65, 65, 65, 65, 0]) -> (x+y=w90:i32[])
            n255 = Byte Array To String(unsigned byte array=w90) -> (string=w80:string)
            n256 = local write "Send String"(w80) -> ()
          }
          frame True {
            # "loop timimng \ncontrolled externally"
            # "embed in loop to left latter"
            # "Send commands to NXT"
            n257 = local read "Mode"() -> (w170:i16)
            n258 = local read "Desired \nVelocity"() -> (w171:i16)
            n259 = local read "Local\nHeading"() -> (w172:i16)
            n260 = Number To Decimal String(number=w170, width (-)=i16 2) -> (decimal integer string=w176:string)
            n261 = Number To Decimal String(number=w171, width (-)=i16 2) -> (decimal integer string=w175:string)
            n262 = Number To Decimal String(number=w172, width (-)=i16 4) -> (decimal integer string=w174:string)
            n263 = Concatenate Strings("$P", w176, w175, w174, "^") -> (w173:string)
            n264 = local write "Send String"(w173) -> ()
          }
        }
        n265 = local read "RunRobot"() -> (w72:bool)
      }
      n266 = while {
        tunnel: w57 -> [_]
        stop <- w187 continue-if-true
        # "Receive information from NXT"
        n267 = local read "String Received"() -> (w192:string)
        n268 = Wait Until Next ms Multiple(millisecond multiple=u32 100) -> ()  [unwired: 1 out]
        n269 = String Subset(string=w192, offset (0)=1, length (rest)=1 ("length (rest)")) -> (substring=w191:string)
        n270 = case shown="\"N\"" w191 {
          tunnel: w192 -> [_ w194]
          frame Default {
          }
          frame "N" {
            # "0-15"
            # "Parse command \"N\""
            n271 = String Subset(string=w194, offset (0)=2, length (rest)=4 ("length (rest)")) -> (substring=w205:string)
            n272 = String Subset(string=w194, offset (0)=6, length (rest)=3 ("length (rest)")) -> (substring=w201:string)
            n273 = String Subset(string=w194, offset (0)=9, length (rest)=2 ("length (rest)")) -> (substring=w197:string)
            n274 = Decimal String To Number(string=w205) -> (number=w208:i32)  [unwired: 2 in, 1 out]
            n275 = Decimal String To Number(string=w201) -> (number=w200:i32)  [unwired: 2 in, 1 out]
            n276 = Decimal String To Number(string=w197) -> (number=w198:i32)  [unwired: 2 in, 1 out]
            n277 = To Word Integer(number=w208) -> (16bit integer=w204:i16)
            n278 = To Word Integer(number=w200) -> (16bit integer=w199:i16)
            n279 = To Long Integer(number=w198) -> (32bit integer=w193:i32)
            n280 = local write "LidarDist"(w199) -> ()
            n281 = local write "Battery\nVolts"(w204) -> ()
            n282 = local write "IR Index"(w193) -> ()
          }
        }
        n283 = local read "RunRobot"() -> (w187:bool)
      }
      n284 = while {
        stop <- w186 continue-if-true
        # "Run Simulated MapDAR"
        n285 = local read "Tug X"() -> (w184:i32)
        n286 = local read "Tug Y"() -> (w183:i32)
        n287 = local read "Tug H"() -> (w182:i32)
        n288 = Bundle "Bundle"("Tug X"=w184, "Tug Y"=w183, "Tug H"=w182) -> (w185:cluster{"Tug X":i32, "Tug Y":i32, "Tug H":i32})  [unwired: 1 in]
        n289 = call "HindbrainLIDAR_Sim.vi"("SubPosition"=w185) -> ("WhatAroundMe?"=→"WhatAroundMeMap?":cluster{"T":dbl, "Range":dbl, "Bearing":dbl}[])  [unwired: 10 in]
        n290 = local read "RunRobot"() -> (w186:bool)
      }
    }
    frame #2 {
      # "Close XBee Radio"
      # "Close UDP port"
      # "Realease LIDAR\nMemory"
      # "Reset Run \nSwitch"
      # "Shutdown Robot"
      n291 = call "Pixel_LIDAR_Close.vi"("error in (no error) 2"=w607, "Image"=w608) -> ()  [unwired: 1 in]
      n292 = local write "RunRobot"(TRUE ("RunRobot")) -> ()
      n293 = call "XB PC Close.vi"("error in (no error)"=w605, "VISA resource name"=w606) -> ()
      n294 = UDP Close(connection ID=w604, 8:w603) -> ()  [unwired: 2 out]
      "error out" <- w605
    }
  }
